vi "GPSPathTrackerTest.vi"() -> ()   [LabVIEW 2024]
uses:
  <vilib>/Instr/_visa.llb/VISA Set IO Buffer Mask.ctl
  <vilib>/Instr/_visa.llb/VISA Flush IO Buffer Mask.ctl
  <vilib>/Utility/file.llb/Read Delimited Spreadsheet (DBL).vi
  <vilib>/Instr/_visa.llb/VISA Configure Serial Port (Instr).vi
panel:
  out "True_Heading(deg)":dbl format="%#_15g"
  out "UTM X(E) INS":dbl format="%#_13g"
  out "UTM Y(N) INS":dbl format="%#_13g"
  out "GPS_Speed(kph)":dbl format="%#_g kph"
  in  "Stop":bool
  out "NMEA_Raw_Data":string
  out "Latitude(deg)":dbl
  out "Logitude(deg)":dbl
  out "Altitude(m)":dbl
  in  "COM7":refnum<visa-resource-name>="COM3" caption="GPS_Com."
  out "Path_lat_arr":dbl[](array[numeric])=[250246.8301, 250246.6716, 250246.4873, 250246.296, 250246.122, 250245.9257, 250245.7732, 250245.5875, 250245.3989, 250245.2166, 250245.0276, 250244.8653, 250244.6749, 250244.5098, 250244.319, 250244.1293, 250243.9404, 250243.757, 250243.5653, 250243.3909, 250243.2171, 250243.0265, 250242.8469, 250242.6561, 250242.4779, 250242.2931, 250242.1112, 250241.9363, 250241.7611, 250241.5908]
  out "Path_long_arr":dbl[](array[numeric])=[3688223.612, 3688223.681, 3688223.731, 3688223.77, 3688223.796, 3688223.82, 3688223.842, 3688223.793, 3688223.791, 3688223.745, 3688223.702, 3688223.665, 3688223.63, 3688223.575, 3688223.538, 3688223.496, 3688223.445, 3688223.39, 3688223.345, 3688223.293, 3688223.242, 3688223.21, 3688223.151, 3688223.108, 3688223.058, 3688223.007, 3688222.954, 3688222.905, 3688222.836, 3688222.787]
  out "Path_Vel_arr":dbl[](array[numeric])=[126.3175841, 126.3175824, 126.3175804, 126.3175784, 126.3175765, 126.3175744, 126.3175727, 126.3175708, 126.3175687, 126.3175668, 126.3175648, 126.3175631, 126.317561, 126.3175593, 126.3175572, 126.3175552, 126.3175532, 126.3175512, 126.3175492, 126.3175473, 126.3175455, 126.3175434, 126.3175415, 126.3175395, 126.3175376, 126.3175356, 126.3175337, 126.3175318, 126.31753, 126.3175282]
  out "Path_Evt_arr":dbl[](array[numeric])=[33.30420584, 33.30420642, 33.30420683, 33.30420714, 33.30420733, 33.3042075, 33.30420766, 33.30420718, 33.30420712, 33.30420667, 33.30420623, 33.30420586, 33.3042055, 33.30420497, 33.30420459, 33.30420417, 33.30420367, 33.30420313, 33.30420267, 33.30420217, 33.30420167, 33.30420133, 33.30420076, 33.30420033, 33.30419983, 33.30419933, 33.30419882, 33.30419833, 33.30419768, 33.30419719]
  out "Evt":dbl
  out "X_lat_path_Full":dbl[](array[numeric])=[250204.6315, 250204.7847, 250204.9423, 250205.0812, 250205.2434, 250205.3871, 250205.5336, 250205.6795, 250205.8333, 250205.974, 250206.1254, 250206.2733, 250206.4155, 250206.5694, 250206.7606, 250206.9331, 250207.0915, 250207.2338, 250207.3801, 250207.5358, 250207.6911, 250207.8385, 250207.9859, 250208.1346, 250208.2889, 250208.4191, 250208.562, 250208.7088, 250208.8428, 250208.9854, 250209.1251, 250209.2579, 250209.3978, 250209.5384, 250209.6838, 250209.8317, 250209.9732, 250210.1069, 250210.2502, 250210.372, 250210.5044, 250210.6376, 250210.7611, 250210.9066, 250211.0503, 250211.1744, 250211.309, 250211.4462, 250211.5776, 250211.7104, 250211.8353, 250211.9552, 250212.0902, 250212.213, 250212.3298, 250212.4572, 250212.5757, 250212.6937, 250212.8209, 250212.9386, 250213.0558, 250213.1735, 250213.2937, 250213.4125, 250213.5502, 250213.6657, 250213.7946, 250213.9274, 250214.0472, 250214.1724, 250214.3017, 250214.4417, 250214.5753, 250214.7017, 250214.8378, 250214.9662, 250215.0894, 250215.2277, 250215.372, 250215.5023, 250215.6465, 250215.6465, 250215.7658, 250215.8914, 250216.017, 250216.142, 250216.2785, 250216.4267, 250216.5776, 250216.7312, 250216.8879, 250217.0506, 250217.2131, 250217.3799, 250217.5426, 250217.7046, 250217.8748, 250218.0423, 250218.2058, 250218.3739, 250218.5355, 250218.7031, 250218.8647, 250219.0346, 250219.1961, 250219.3482, 250219.5145, 250219.672, 250219.8212, 250219.9767, 250220.1301, 250220.2837, 250220.4332, 250220.5777, 250220.7226, 250220.8672, 250221.0139, 250221.1635, 250221.2913, 250221.4361, 250221.5854, 250221.7202, 250221.862, 250222.0043, 250222.1442, 250222.2947, 250222.4297, 250222.5803, 250222.7124, 250222.8553, 250222.9875, 250223.1252, 250223.2779, 250223.409, 250223.5472, 250223.6863, 250223.8257, 250223.9601, 250224.1026, 250224.2408, 250224.3821, 250224.528, 250224.675, 250224.8272, 250224.9781, 250225.124, 250225.2738, 250225.4183, 250225.5696, 250225.7148, 250225.8666, 250226.0158, 250226.1696, 250226.314, 250226.464, 250226.616, 250226.7669, 250226.8995, 250227.0551, 250227.2017, 250227.3491, 250227.4987, 250227.651, 250227.8032, 250227.9491, 250228.1012, 250228.2468, 250228.3977, 250228.5421, 250228.6906, 250228.8411, 250228.9881, 250229.1171, 250229.2733, 250229.4177, 250229.5665, 250229.7135, 250229.8553, 250229.9955, 250230.1399, 250230.2778, 250230.4184, 250230.5592, 250230.6982, 250230.8426, 250230.9741, 250231.1183, 250231.2583, 250231.3917, 250231.5316, 250231.664, 250231.809, 250231.9365, 250232.0794, 250232.2326, 250232.3781, 250232.5288, 250232.6849, 250232.849, 250233.0169, 250233.1898, 250233.3618, 250233.5347, 250233.7129, 250233.8854, 250234.0582, 250234.2271, 250234.392, 250234.5465, 250234.6882, 250234.8252, 250234.962, 250235.0951, 250235.2304, 250235.3491, 250235.4717, 250235.6036, 250235.7176, 250235.8287, 250235.9455, 250236.054, 250236.1492, 250236.2337, 250236.312, 250236.3794, 250236.4369, 250236.4842, 250236.5555, 250236.5952, 250236.6264, 250236.6586, 250236.6755, 250236.6895, 250236.6942, 250236.697, 250236.6851, 250236.6654, 250236.6292, 250236.5933, 250236.551, 250236.4843, 250236.4291, 250236.3642, 250236.3049, 250236.2381, 250236.1715, 250236.0948, 250236.0356, 250235.9406, 250235.8714, 250235.7898, 250235.7058, 250235.658, 250235.5758, 250235.4943, 250235.4193, 250235.3767, 250235.3402, 250235.2889, 250235.2668, 250235.2332, 250235.1891, 250235.1614, 250235.1565, 250235.1204, 250235.1167, 250235.133, 250235.1628, 250235.1974, 250235.2612, 250235.3531, 250235.4155, 250235.5356, 250235.6584, 250235.7924, 250235.9326, 250236.0835, 250236.1855, 250236.3061, 250236.46, 250236.5583, 250236.7204, 250236.8858, 250237.0619, 250237.2443, 250237.4126, 250237.579, 250237.7347, 250237.9052, 250238.0628, 250238.1948, 250238.3334, 250238.4969, 250238.6626, 250238.831, 250239.0118, 250239.1778, 250239.3373, 250239.5311, 250239.6876, 250239.8513, 250240.05, 250240.2334, 250240.4321, 250240.6256, 250240.816, 250240.9998, 250241.1899, 250241.3681, 250241.5524, 250241.7339, 250241.9189, 250242.1048, 250242.2826, 250242.4514, 250242.6353, 250242.8115, 250242.986, 250243.1671, 250243.3465, 250243.5187, 250243.6972, 250243.888, 250244.084, 250244.2833, 250244.4766, 250244.6711, 250244.8658, 250245.0556, 250245.2439, 250245.4299, 250245.6119, 250245.7785, 250245.9451, 250246.096, 250246.2496, 250246.3875, 250246.5144, 250246.631, 250246.7342, 250246.8204, 250246.907, 250247.0092, 250247.1016, 250247.193, 250247.2639, 250247.3441, 250247.421, 250247.4764, 250247.5347, 250247.5768, 250247.6199, 250247.652, 250247.665, 250247.6714, 250247.6666, 250247.6394, 250247.6096, 250247.5413, 250247.498, 250247.4546, 250247.3884, 250247.3334, 250247.2883, 250247.2288, 250247.1836, 250247.1639, 250247.1466, 250247.1079, 250247.1021, 250247.0827, 250247.0531, 250247.0114, 250247.0067, 250246.9862, 250246.9811, 250246.9938, 250247.0308, 250247.0702, 250247.135, 250247.2146, 250247.3014, 250247.4225, 250247.5588, 250247.6858, 250247.828, 250247.9565, 250248.126, 250248.2664, 250248.409, 250248.5611, 250248.7068, 250248.8531, 250249.0229, 250249.202, 250249.3857, 250249.5753, 250249.7637, 250249.959, 250250.1426, 250250.3367, 250250.5143, 250250.6887, 250250.882, 250251.0751, 250251.2683, 250251.4599, 250251.6407, 250251.8269, 250252.0222, 250252.215, 250252.3883, 250252.58, 250252.7757, 250252.9624, 250253.1529, 250253.3403, 250253.5294, 250253.7184, 250253.907, 250254.0796, 250254.2588, 250254.4147, 250254.5819, 250254.743, 250254.8895, 250255.0112, 250255.1568, 250255.2877, 250255.437, 250255.5889, 250255.7462, 250255.9147, 250256.0842, 250256.2597, 250256.4476, 250256.6251, 250256.814, 250257.0016, 250257.1907, 250257.383, 250257.5732, 250257.7644, 250257.9556, 250258.1438, 250258.3228, 250258.5095, 250258.6883, 250258.8678, 250259.0368, 250259.2086, 250259.3646, 250259.5205, 250259.6669, 250259.7981, 250259.9204, 250260.0341, 250260.1304, 250260.2154, 250260.2683, 250260.3212, 250260.3713, 250260.4074, 250260.4278, 250260.4483, 250260.4538, 250260.4584, 250260.4638, 250260.4531, 250260.4269, 250260.4025, 250260.3748, 250260.3569, 250260.3259, 250260.306, 250260.3019, 250260.2913, 250260.2964, 250260.3013, 250260.322, 250260.3442, 250260.3803, 250260.414, 250260.462, 250260.5251, 250260.6072, 250260.6942, 250260.7672, 250260.8711, 250260.9697, 250261.0724, 250261.1817, 250261.2963, 250261.3941, 250261.4821, 250261.569, 250261.6706, 250261.7652, 250261.857, 250261.9183, 250261.9427, 250261.9912, 250261.9961, 250262.0007, 250261.9756, 250261.9489, 250261.9099, 250261.8812, 250261.8445, 250261.7817, 250261.7129, 250261.6398, 250261.5329, 250261.4604, 250261.3434, 250261.24, 250261.1259, 250260.9928, 250260.8741, 250260.7678, 250260.6137, 250260.4623, 250260.2939, 250260.126, 250259.9411, 250259.7546, 250259.5669, 250259.4199, 250259.2239, 250259.0425, 250258.8499, 250258.6584, 250258.475, 250258.2939, 250258.1037, 250257.9137, 250257.7231, 250257.5553, 250257.3716, 250257.2069, 250257.0301, 250256.8666, 250256.6854, 250256.514, 250256.3482, 250256.1782, 250256.0288, 250255.8463, 250255.6842, 250255.5166, 250255.3463, 250255.1982, 250255.0421, 250254.892, 250254.7261, 250254.5713, 250254.4091, 250254.2573, 250254.0995, 250253.9355, 250253.7624, 250253.5867, 250253.3985, 250253.2139, 250253.0287, 250252.8354, 250252.6448, 250252.4492, 250252.2513, 250252.0571, 250251.8685, 250251.6866, 250251.5105, 250251.3443, 250251.1824, 250251.0309, 250250.8789, 250250.7367, 250250.5995, 250250.4539, 250250.3121, 250250.1719, 250250.0299, 250249.887, 250249.7463, 250249.6052, 250249.4649, 250249.331, 250249.1893, 250249.0528, 250248.9386, 250248.8243, 250248.7236, 250248.6306, 250248.529, 250248.4359, 250248.3517, 250248.2827, 250248.2037, 250248.1463, 250248.0957, 250248.0509, 250248.0219, 250248.0051, 250247.9945, 250247.9837, 250247.989, 250247.9941, 250247.9993, 250248.0044, 250248.0095, 250248.0145, 250248.0352, 250248.0557, 250248.0919, 250248.1148, 250248.1615, 250248.1868, 250248.2214, 250248.2728, 250248.3179, 250248.3416, 250248.3511, 250248.3839, 250248.4042, 250248.432, 250248.4459, 250248.4908, 250248.5037, 250248.5435, 250248.5875, 250248.6237, 250248.6436, 250248.6662, 250248.6992, 250248.705, 250248.7258, 250248.7267, 250248.7214, 250248.7308, 250248.744, 250248.7337, 250248.7226, 250248.6855, 250248.6674, 250248.5843, 250248.537, 250248.448, 250248.3765, 250248.2712, 250248.1941, 250248.1144, 250247.9992, 250247.891, 250247.7807, 250247.6307, 250247.5171, 250247.3602, 250247.1874, 250247.0166, 250246.8301, 250246.6716, 250246.4873, 250246.296, 250246.122, 250245.9257, 250245.7732, 250245.5875, 250245.3989, 250245.2166, 250245.0276, 250244.8653, 250244.6749, 250244.5098, 250244.319, 250244.1293, 250243.9404, 250243.757, 250243.5653, 250243.3909, 250243.2171, 250243.0265, 250242.8469, 250242.6561, 250242.4779, 250242.2931, 250242.1112, 250241.9363, 250241.7611, 250241.5908, 250241.4105, 250241.2326, 250241.0415, 250240.8823, 250240.7086, 250240.5237, 250240.3385, 250240.1546, 250239.9595, 250239.7651, 250239.5694, 250239.3713, 250239.1737, 250238.9795, 250238.7874, 250238.5977, 250238.4158, 250238.2247, 250238.0451, 250237.867, 250237.6942, 250237.5189, 250237.359, 250237.1898, 250237.0315, 250236.8728, 250236.7137, 250236.5718, 250236.437, 250236.2994, 250236.1879, 250236.0639, 250235.9389, 250235.83, 250235.7229, 250235.6297, 250235.5351, 250235.4494, 250235.3697, 250235.3065, 250235.2435, 250235.1994, 250235.1375, 250235.0894, 250235.041, 250235.0127, 250234.9717, 250234.9373, 250234.9195, 250234.8912, 250234.852, 250234.8256, 250234.8066, 250234.7894, 250234.7971, 250234.798, 250234.7875, 250234.8083, 250234.8039, 250234.8027, 250234.8079, 250234.813, 250234.8181, 250234.8119, 250234.8202, 250234.8152, 250234.8222, 250234.8216, 250234.7975, 250234.7903, 250234.7485, 250234.7087, 250234.6504, 250234.616, 250234.567, 250234.5014, 250234.4497, 250234.3789, 250234.3334, 250234.2602, 250234.1655, 250234.0706, 250233.9596, 250233.8482, 250233.6928, 250233.5374, 250233.4092, 250233.2698, 250233.1115, 250232.9573, 250232.785, 250232.598, 250232.4051, 250232.2295, 250232.0509, 250231.866, 250231.6857, 250231.4995, 250231.3134, 250231.1433, 250230.9457, 250230.7492, 250230.5768, 250230.3831, 250230.1894, 250229.9975, 250229.8111, 250229.6241, 250229.4384, 250229.2517, 250229.069, 250228.8781, 250228.6895, 250228.511, 250228.3291, 250228.1418, 250227.9599, 250227.7698, 250227.597, 250227.4079, 250227.2175, 250227.0293, 250226.8363, 250226.6397, 250226.4445, 250226.4445, 250226.3195, 250226.1946, 250226.0696, 250225.9221, 250225.7742, 250225.6168, 250225.47, 250225.3233, 250225.1765, 250225.0287, 250224.8822, 250224.7443, 250224.5996, 250224.4528, 250224.301, 250224.1558, 250224.0269, 250223.8866, 250223.7351, 250223.5855, 250223.4444, 250223.2886, 250223.148, 250223.0104, 250222.8695, 250222.7295, 250222.5838, 250222.4554, 250222.316, 250222.1912, 250222.056, 250221.9297, 250221.7922, 250221.6642, 250221.5466, 250221.3995, 250221.2768, 250221.1432, 250221.0095, 250220.8891, 250220.7597, 250220.6502, 250220.5287, 250220.4116, 250220.2851, 250220.1647, 250220.0444, 250219.9261, 250219.7966, 250219.6741, 250219.5628, 250219.4354, 250219.3182, 250219.1887, 250219.0582, 250218.9251, 250218.8036, 250218.679, 250218.5495, 250218.4169, 250218.2866, 250218.1513, 250218.0199, 250217.8896, 250217.7568, 250217.6185, 250217.4845, 250217.3551, 250217.2166, 250217.0853, 250216.9453, 250216.8055, 250216.6585, 250216.5131, 250216.3689, 250216.2118, 250216.0655, 250215.9129, 250215.7606, 250215.6071, 250215.4505, 250215.2942, 250215.1411, 250214.9841, 250214.842, 250214.6871, 250214.5483, 250214.3987, 250214.2557, 250214.1195, 250213.9747, 250213.8377, 250213.7044, 250213.5703, 250213.4445, 250213.3184, 250213.183, 250213.0559, 250212.9317, 250212.8112, 250212.6789, 250212.5512, 250212.4267, 250212.2918, 250212.1645, 250212.0429, 250211.9046, 250211.769, 250211.6308, 250211.492, 250211.3609, 250211.2259, 250211.0952, 250210.9578, 250210.8141, 250210.6818, 250210.5388, 250210.4096, 250210.2669, 250210.1265, 250209.986, 250209.8443, 250209.696, 250209.5582, 250209.4275, 250209.2882, 250209.1319, 250209.0284]
  out "vel. path":dbl[](array[numeric])=[126.317125, 126.3171267, 126.3171284, 126.3171299, 126.3171317, 126.3171333, 126.3171349, 126.3171365, 126.3171382, 126.3171397, 126.3171414, 126.317143, 126.3171446, 126.3171463, 126.3171483, 126.3171502, 126.317152, 126.3171535, 126.3171551, 126.3171568, 126.3171585, 126.3171601, 126.3171618, 126.3171634, 126.3171651, 126.3171665, 126.3171681, 126.3171697, 126.3171712, 126.3171728, 126.3171743, 126.3171758, 126.3171773, 126.3171788, 126.3171804, 126.3171821, 126.3171836, 126.3171851, 126.3171867, 126.317188, 126.3171895, 126.317191, 126.3171923, 126.3171939, 126.3171955, 126.3171969, 126.3171984, 126.3171999, 126.3172013, 126.3172028, 126.3172042, 126.3172055, 126.317207, 126.3172083, 126.3172096, 126.3172111, 126.3172124, 126.3172137, 126.3172151, 126.3172164, 126.3172177, 126.317219, 126.3172203, 126.3172217, 126.3172232, 126.3172245, 126.3172259, 126.3172273, 126.3172287, 126.3172301, 126.3172315, 126.317233, 126.3172345, 126.3172359, 126.3172374, 126.3172388, 126.3172402, 126.3172417, 126.3172433, 126.3172447, 126.3172463, 126.3172463, 126.3172476, 126.317249, 126.3172504, 126.3172518, 126.3172533, 126.3172549, 126.3172566, 126.3172583, 126.31726, 126.3172618, 126.3172635, 126.3172654, 126.3172671, 126.3172689, 126.3172708, 126.3172726, 126.3172744, 126.3172762, 126.317278, 126.3172798, 126.3172816, 126.3172834, 126.3172852, 126.3172868, 126.3172886, 126.3172904, 126.317292, 126.3172937, 126.3172954, 126.3172971, 126.3172987, 126.3173003, 126.3173019, 126.3173035, 126.3173051, 126.3173067, 126.3173081, 126.3173097, 126.3173114, 126.3173129, 126.3173144, 126.317316, 126.3173175, 126.3173192, 126.3173207, 126.3173223, 126.3173238, 126.3173253, 126.3173268, 126.3173283, 126.31733, 126.3173314, 126.317333, 126.3173345, 126.317336, 126.3173375, 126.3173391, 126.3173406, 126.3173421, 126.3173437, 126.3173454, 126.317347, 126.3173487, 126.3173503, 126.3173519, 126.3173535, 126.3173552, 126.3173568, 126.3173584, 126.3173601, 126.3173617, 126.3173633, 126.317365, 126.3173666, 126.3173683, 126.3173698, 126.3173715, 126.3173731, 126.3173747, 126.3173763, 126.317378, 126.3173797, 126.3173813, 126.3173829, 126.3173845, 126.3173862, 126.3173878, 126.3173894, 126.3173911, 126.3173927, 126.3173941, 126.3173958, 126.3173974, 126.317399, 126.3174006, 126.3174022, 126.3174037, 126.3174053, 126.3174068, 126.3174084, 126.3174099, 126.3174115, 126.3174131, 126.3174145, 126.3174161, 126.3174176, 126.3174191, 126.3174206, 126.3174221, 126.3174237, 126.3174251, 126.3174267, 126.3174284, 126.31743, 126.3174316, 126.3174333, 126.3174351, 126.3174369, 126.3174388, 126.3174407, 126.3174426, 126.3174445, 126.3174464, 126.3174483, 126.3174501, 126.3174519, 126.3174536, 126.3174552, 126.3174567, 126.3174582, 126.3174596, 126.3174611, 126.3174624, 126.3174638, 126.3174653, 126.3174665, 126.3174678, 126.3174691, 126.3174703, 126.3174713, 126.3174723, 126.3174732, 126.317474, 126.3174746, 126.3174752, 126.317476, 126.3174765, 126.3174769, 126.3174773, 126.3174775, 126.3174777, 126.3174778, 126.3174779, 126.3174778, 126.3174777, 126.3174773, 126.317477, 126.3174766, 126.3174759, 126.3174754, 126.3174748, 126.3174742, 126.3174735, 126.3174728, 126.3174721, 126.3174715, 126.3174705, 126.3174698, 126.317469, 126.3174681, 126.3174677, 126.3174668, 126.317466, 126.3174653, 126.3174648, 126.3174645, 126.317464, 126.3174638, 126.3174635, 126.3174631, 126.3174628, 126.3174628, 126.3174625, 126.3174625, 126.3174627, 126.3174631, 126.3174635, 126.3174643, 126.3174653, 126.317466, 126.3174673, 126.3174687, 126.3174702, 126.3174717, 126.3174734, 126.3174745, 126.3174758, 126.3174775, 126.31747849999999, 126.3174803, 126.3174821, 126.317484, 126.317486, 126.3174878, 126.3174896, 126.3174913, 126.3174932, 126.3174949, 126.3174963, 126.3174978, 126.3174996, 126.3175014, 126.3175032, 126.3175052, 126.317507, 126.3175087, 126.3175108, 126.3175125, 126.3175142, 126.3175164, 126.3175183, 126.3175205, 126.3175225, 126.3175246, 126.3175265, 126.3175286, 126.3175305, 126.3175324, 126.3175344, 126.3175363, 126.3175383, 126.3175402, 126.317542, 126.3175439, 126.3175458, 126.3175477, 126.3175496, 126.3175515, 126.3175533, 126.3175552, 126.3175573, 126.3175594, 126.3175615, 126.3175636, 126.3175657, 126.3175678, 126.3175698, 126.3175719, 126.3175739, 126.3175759, 126.3175777, 126.3175795, 126.3175811, 126.3175828, 126.3175843, 126.3175857, 126.317587, 126.3175882, 126.3175892, 126.3175901, 126.3175913, 126.3175923, 126.3175933, 126.3175942, 126.3175951, 126.3175959, 126.3175966, 126.3175973, 126.3175978, 126.3175983, 126.3175987, 126.3175989, 126.317599, 126.317599, 126.3175988, 126.3175985, 126.3175978, 126.3175974, 126.317597, 126.3175963, 126.3175958, 126.3175954, 126.3175948, 126.3175943, 126.3175942, 126.317594, 126.3175937, 126.3175937, 126.3175935, 126.3175932, 126.3175928, 126.3175928, 126.3175927, 126.3175927, 126.3175929, 126.3175933, 126.3175938, 126.3175945, 126.3175954, 126.3175964, 126.3175977, 126.3175992, 126.3176006, 126.3176022, 126.3176036, 126.3176055, 126.317607, 126.3176086, 126.3176102, 126.3176118, 126.3176134, 126.3176152, 126.3176172, 126.3176192, 126.3176212, 126.3176233, 126.3176254, 126.3176274, 126.3176294, 126.3176314, 126.3176333, 126.3176353, 126.3176374, 126.3176395, 126.3176416, 126.3176435, 126.3176455, 126.3176476, 126.3176497, 126.3176515, 126.3176536, 126.3176557, 126.3176577, 126.3176597, 126.3176617, 126.3176637, 126.3176657, 126.3176677, 126.3176696, 126.3176715, 126.3176731, 126.3176749, 126.3176766, 126.3176781, 126.3176794, 126.3176809, 126.3176823, 126.3176838, 126.3176854, 126.3176871, 126.3176889, 126.3176906, 126.3176925, 126.3176945, 126.3176964, 126.3176984, 126.3177004, 126.3177024, 126.3177044, 126.3177065, 126.3177085, 126.3177106, 126.3177126, 126.3177145, 126.3177164, 126.3177183, 126.3177202, 126.317722, 126.3177238, 126.3177255, 126.3177271, 126.3177287, 126.31773, 126.3177313, 126.3177325, 126.3177335, 126.3177343, 126.3177348, 126.3177353, 126.3177358, 126.3177362, 126.3177363, 126.3177365, 126.3177365, 126.3177365, 126.3177365, 126.3177363, 126.317736, 126.3177357, 126.3177353, 126.3177351, 126.3177347, 126.3177344, 126.3177343, 126.3177342, 126.3177342, 126.3177342, 126.3177343, 126.3177345, 126.3177349, 126.3177352, 126.3177356, 126.3177362, 126.3177371, 126.317738, 126.3177387, 126.3177398, 126.3177408, 126.3177418, 126.317743, 126.3177441, 126.3177452, 126.317746, 126.3177469, 126.317748, 126.3177489, 126.3177499, 126.3177505, 126.3177507, 126.3177512, 126.3177512, 126.3177512, 126.3177508, 126.3177505, 126.31775, 126.3177497, 126.3177492, 126.3177485, 126.3177477, 126.3177469, 126.3177457, 126.3177449, 126.3177436, 126.3177424, 126.3177412, 126.3177397, 126.3177384, 126.3177372, 126.3177355, 126.3177339, 126.317732, 126.3177302, 126.3177282, 126.3177262, 126.3177242, 126.3177226, 126.3177205, 126.3177186, 126.3177165, 126.3177145, 126.3177125, 126.3177106, 126.3177085, 126.3177065, 126.3177045, 126.3177027, 126.3177007, 126.317699, 126.3176971, 126.3176954, 126.3176934, 126.3176916, 126.3176899, 126.3176881, 126.3176865, 126.3176845, 126.3176828, 126.3176811, 126.3176793, 126.3176777, 126.317676, 126.3176745, 126.3176727, 126.3176711, 126.3176694, 126.3176678, 126.3176661, 126.3176644, 126.3176626, 126.3176607, 126.3176587, 126.3176567, 126.3176548, 126.3176527, 126.3176507, 126.3176486, 126.3176464, 126.3176444, 126.3176423, 126.3176403, 126.3176384, 126.3176366, 126.3176349, 126.3176332, 126.3176315, 126.31763, 126.3176285, 126.3176269, 126.3176253, 126.3176238, 126.3176222, 126.3176206, 126.3176191, 126.3176175, 126.317616, 126.3176145, 126.3176129, 126.3176114, 126.3176102, 126.3176089, 126.3176078, 126.3176067, 126.3176056, 126.3176045, 126.3176036, 126.3176028, 126.3176019, 126.3176012, 126.3176006, 126.3176001, 126.3175997, 126.3175995, 126.3175993, 126.3175992, 126.3175992, 126.3175992, 126.3175992, 126.3175992, 126.3175992, 126.3175992, 126.3175993, 126.3175995, 126.3175998, 126.3176, 126.3176005, 126.3176007, 126.317601, 126.3176015, 126.3176019, 126.3176022, 126.3176022, 126.3176025, 126.3176027, 126.3176029, 126.317603, 126.3176034, 126.3176035, 126.3176039, 126.3176043, 126.3176047, 126.3176048, 126.317605, 126.3176053, 126.3176053, 126.3176055, 126.3176055, 126.3176054, 126.3176054, 126.3176055, 126.3176053, 126.3176052, 126.3176047, 126.3176045, 126.3176035, 126.317603, 126.317602, 126.3176012, 126.3176, 126.3175991, 126.3175982, 126.3175969, 126.3175957, 126.3175945, 126.3175929, 126.3175916, 126.3175899, 126.317588, 126.3175862, 126.3175841, 126.3175824, 126.3175804, 126.3175784, 126.3175765, 126.3175744, 126.3175727, 126.3175708, 126.3175687, 126.3175668, 126.3175648, 126.3175631, 126.317561, 126.3175593, 126.3175572, 126.3175552, 126.3175532, 126.3175512, 126.3175492, 126.3175473, 126.3175455, 126.3175434, 126.3175415, 126.3175395, 126.3175376, 126.3175356, 126.3175337, 126.3175318, 126.31753, 126.3175282, 126.3175262, 126.3175243, 126.3175223, 126.3175206, 126.3175188, 126.3175168, 126.3175148, 126.3175129, 126.3175108, 126.3175087, 126.3175066, 126.3175045, 126.3175024, 126.3175003, 126.3174982, 126.3174961, 126.3174942, 126.3174921, 126.3174902, 126.3174882, 126.3174863, 126.3174844, 126.3174827, 126.3174809, 126.3174791, 126.3174774, 126.3174756, 126.3174741, 126.3174726, 126.3174711, 126.3174698, 126.3174685, 126.3174671, 126.3174659, 126.3174647, 126.3174636, 126.3174626, 126.3174616, 126.3174607, 126.31746, 126.3174592, 126.3174587, 126.317458, 126.3174574, 126.3174568, 126.3174565, 126.317456, 126.3174556, 126.3174553, 126.317455, 126.3174545, 126.3174542, 126.3174539, 126.3174537, 126.3174537, 126.3174537, 126.3174535, 126.3174537, 126.3174536, 126.3174535, 126.3174535, 126.3174535, 126.3174535, 126.3174534, 126.3174534, 126.3174533, 126.3174533, 126.3174533, 126.317453, 126.3174528, 126.3174523, 126.3174519, 126.3174512, 126.3174508, 126.3174502, 126.3174494, 126.3174488, 126.317448, 126.3174475, 126.3174467, 126.3174456, 126.3174445, 126.3174433, 126.3174421, 126.3174404, 126.3174387, 126.3174373, 126.3174358, 126.317434, 126.3174324, 126.3174305, 126.3174285, 126.3174264, 126.3174245, 126.3174226, 126.3174206, 126.3174187, 126.3174167, 126.3174147, 126.3174128, 126.3174107, 126.3174086, 126.3174068, 126.3174047, 126.3174026, 126.3174006, 126.3173986, 126.3173966, 126.3173946, 126.3173926, 126.3173907, 126.3173887, 126.3173867, 126.3173848, 126.3173828, 126.3173808, 126.3173789, 126.3173769, 126.317375, 126.317373, 126.317371, 126.317369, 126.3173669, 126.31736480000001, 126.3173627, 126.3173627, 126.3173614, 126.31736, 126.3173587, 126.3173571, 126.3173554, 126.3173537, 126.3173521, 126.3173505, 126.3173489, 126.3173473, 126.3173457, 126.3173441, 126.3173426, 126.3173409, 126.3173393, 126.3173377, 126.3173363, 126.3173347, 126.3173331, 126.3173314, 126.3173299, 126.3173282, 126.3173266, 126.3173251, 126.3173235, 126.317322, 126.3173204, 126.317319, 126.3173175, 126.3173161, 126.3173146, 126.3173132, 126.3173117, 126.3173103, 126.3173089, 126.3173073, 126.317306, 126.3173045, 126.317303, 126.3173017, 126.3173003, 126.317299, 126.3172977, 126.3172964, 126.317295, 126.3172937, 126.3172923, 126.317291, 126.3172896, 126.3172882, 126.317287, 126.3172856, 126.3172843, 126.3172829, 126.3172814, 126.31728, 126.3172786, 126.3172772, 126.3172758, 126.3172743, 126.3172729, 126.3172714, 126.31727, 126.3172685, 126.317267, 126.3172655, 126.317264, 126.3172626, 126.3172611, 126.3172596, 126.3172581, 126.3172566, 126.317255, 126.3172534, 126.3172518, 126.3172501, 126.3172485, 126.3172468, 126.3172451, 126.3172434, 126.3172417, 126.31724, 126.3172383, 126.3172366, 126.3172351, 126.3172334, 126.3172318, 126.3172302, 126.3172286, 126.3172271, 126.3172255, 126.317224, 126.3172225, 126.3172211, 126.3172197, 126.3172183, 126.3172168, 126.3172154, 126.317214, 126.3172127, 126.3172112, 126.3172098, 126.3172084, 126.3172069, 126.3172055, 126.3172042, 126.3172027, 126.3172012, 126.3171997, 126.3171981, 126.3171967, 126.3171952, 126.3171937, 126.3171922, 126.3171907, 126.3171892, 126.3171876, 126.3171862, 126.3171846, 126.3171831, 126.3171815, 126.31718, 126.3171783, 126.3171768, 126.3171754, 126.3171739, 126.3171721, 126.317171]
  out "Y_long_path_Full":dbl[](array[numeric])=[3688246.636, 3688246.509, 3688246.386, 3688246.252, 3688246.131, 3688245.999, 3688245.863, 3688245.725, 3688245.593, 3688245.45, 3688245.315, 3688245.179, 3688245.039, 3688244.911, 3688244.843, 3688244.735, 3688244.608, 3688244.485, 3688244.347, 3688244.225, 3688244.098, 3688243.962, 3688243.826, 3688243.702, 3688243.576, 3688243.428, 3688243.289, 3688243.152, 3688243.019, 3688242.881, 3688242.758, 3688242.611, 3688242.466, 3688242.324, 3688242.184, 3688242.046, 3688241.912, 3688241.761, 3688241.621, 3688241.464, 3688241.317, 3688241.168, 3688241.016, 3688240.878, 3688240.743, 3688240.587, 3688240.445, 3688240.302, 3688240.154, 3688240.007, 3688239.85, 3688239.697, 3688239.549, 3688239.391, 3688239.229, 3688239.078, 3688238.919, 3688238.759, 3688238.606, 3688238.449, 3688238.288, 3688238.132, 3688237.972, 3688237.812, 3688237.667, 3688237.509, 3688237.359, 3688237.212, 3688237.056, 3688236.903, 3688236.761, 3688236.618, 3688236.472, 3688236.318, 3688236.18, 3688236.04, 3688235.882, 3688235.736, 3688235.602, 3688235.455, 3688235.317, 3688235.317, 3688235.161, 3688235.009, 3688234.859, 3688234.707, 3688234.563, 3688234.431, 3688234.301, 3688234.177, 3688234.058, 3688233.945, 3688233.832, 3688233.726, 3688233.616, 3688233.504, 3688233.406, 3688233.302, 3688233.192, 3688233.09, 3688232.98, 3688232.875, 3688232.767, 3688232.663, 3688232.554, 3688232.429, 3688232.322, 3688232.207, 3688232.075, 3688231.951, 3688231.826, 3688231.702, 3688231.575, 3688231.444, 3688231.311, 3688231.182, 3688231.047, 3688230.919, 3688230.774, 3688230.641, 3688230.511, 3688230.367, 3688230.231, 3688230.094, 3688229.957, 3688229.829, 3688229.683, 3688229.557, 3688229.413, 3688229.278, 3688229.132, 3688228.991, 3688228.865, 3688228.717, 3688228.577, 3688228.436, 3688228.296, 3688228.16, 3688228.023, 3688227.884, 3688227.749, 3688227.618, 3688227.486, 3688227.365, 3688227.239, 3688227.103, 3688226.975, 3688226.839, 3688226.711, 3688226.574, 3688226.45, 3688226.318, 3688226.199, 3688226.063, 3688225.934, 3688225.812, 3688225.684, 3688225.54, 3688225.421, 3688225.29, 3688225.156, 3688225.028, 3688224.9, 3688224.772, 3688224.642, 3688224.516, 3688224.383, 3688224.257, 3688224.124, 3688223.994, 3688223.865, 3688223.735, 3688223.59, 3688223.474, 3688223.338, 3688223.207, 3688223.074, 3688222.936, 3688222.795, 3688222.659, 3688222.518, 3688222.382, 3688222.244, 3688222.105, 3688221.97, 3688221.825, 3688221.694, 3688221.554, 3688221.407, 3688221.266, 3688221.121, 3688220.986, 3688220.837, 3688220.7, 3688220.579, 3688220.446, 3688220.321, 3688220.2, 3688220.09, 3688219.984, 3688219.886, 3688219.791, 3688219.695, 3688219.609, 3688219.511, 3688219.412, 3688219.312, 3688219.202, 3688219.08, 3688218.943, 3688218.802, 3688218.658, 3688218.514, 3688218.373, 3688218.215, 3688218.06, 3688217.916, 3688217.752, 3688217.592, 3688217.434, 3688217.271, 3688217.096, 3688216.918, 3688216.738, 3688216.555, 3688216.364, 3688216.175, 3688215.99, 3688215.797, 3688215.603, 3688215.408, 3688215.212, 3688215.018, 3688214.825, 3688214.629, 3688214.435, 3688214.238, 3688214.045, 3688213.854, 3688213.659, 3688213.473, 3688213.282, 3688213.096, 3688212.911, 3688212.732, 3688212.553, 3688212.373, 3688212.187, 3688212.026, 3688211.845, 3688211.666, 3688211.498, 3688211.307, 3688211.137, 3688210.957, 3688210.774, 3688210.583, 3688210.455, 3688210.27, 3688210.079, 3688209.89, 3688209.707, 3688209.511, 3688209.32, 3688209.133, 3688208.944, 3688208.778, 3688208.603, 3688208.425, 3688208.24, 3688208.069, 3688207.923, 3688207.776, 3688207.638, 3688207.505, 3688207.376, 3688207.261, 3688207.163, 3688207.105, 3688206.993, 3688206.89, 3688206.843, 3688206.777, 3688206.715, 3688206.655, 3688206.559, 3688206.461, 3688206.366, 3688206.273, 3688206.184, 3688206.113, 3688205.99, 3688205.895, 3688205.827, 3688205.775, 3688205.706, 3688205.658, 3688205.603, 3688205.616, 3688205.607, 3688205.608, 3688205.602, 3688205.579, 3688205.574, 3688205.595, 3688205.626, 3688205.67, 3688205.702, 3688205.765, 3688205.832, 3688205.892, 3688205.924, 3688205.975, 3688206.044, 3688206.125, 3688206.183, 3688206.249, 3688206.333, 3688206.409, 3688206.446, 3688206.526, 3688206.566, 3688206.595, 3688206.609, 3688206.603, 3688206.58, 3688206.556, 3688206.533, 3688206.491, 3688206.441, 3688206.381, 3688206.31, 3688206.213, 3688206.118, 3688205.996, 3688205.876, 3688205.735, 3688205.585, 3688205.428, 3688205.261, 3688205.087, 3688204.913, 3688204.745, 3688204.572, 3688204.399, 3688204.217, 3688204.041, 3688203.86, 3688203.671, 3688203.482, 3688203.291, 3688203.097, 3688202.903, 3688202.706, 3688202.51, 3688202.313, 3688202.121, 3688201.928, 3688201.742, 3688201.55, 3688201.357, 3688201.175, 3688201.009, 3688200.831, 3688200.66, 3688200.469, 3688200.293, 3688200.102, 3688199.927, 3688199.75, 3688199.553, 3688199.364, 3688199.207, 3688199.015, 3688198.819, 3688198.62, 3688198.43, 3688198.239, 3688198.051, 3688197.866, 3688197.706, 3688197.53, 3688197.389, 3688197.254, 3688197.113, 3688197.004, 3688196.877, 3688196.777, 3688196.671, 3688196.564, 3688196.467, 3688196.356, 3688196.256, 3688196.178, 3688196.107, 3688196.03, 3688195.977, 3688195.933, 3688195.904, 3688195.84, 3688195.809, 3688195.77, 3688195.714, 3688195.686, 3688195.663, 3688195.635, 3688195.597, 3688195.593, 3688195.569, 3688195.582, 3688195.578, 3688195.592, 3688195.622, 3688195.638, 3688195.688, 3688195.721, 3688195.771, 3688195.83, 3688195.888, 3688195.924, 3688196.013, 3688196.097, 3688196.199, 3688196.297, 3688196.407, 3688196.538, 3688196.689, 3688196.822, 3688196.969, 3688197.098, 3688197.223, 3688197.336, 3688197.437, 3688197.537, 3688197.627, 3688197.689, 3688197.772, 3688197.835, 3688197.898, 3688197.962, 3688198.006, 3688198.066, 3688198.118, 3688198.16, 3688198.22, 3688198.3, 3688198.363, 3688198.445, 3688198.523, 3688198.622, 3688198.722, 3688198.834, 3688198.951, 3688199.084, 3688199.233, 3688199.389, 3688199.552, 3688199.724, 3688199.899, 3688200.09, 3688200.276, 3688200.466, 3688200.659, 3688200.855, 3688201.049, 3688201.243, 3688201.442, 3688201.641, 3688201.837, 3688202.031, 3688202.224, 3688202.419, 3688202.615, 3688202.809, 3688203.003, 3688203.2, 3688203.398, 3688203.596, 3688203.795, 3688203.99, 3688204.187, 3688204.382, 3688204.576, 3688204.768, 3688204.955, 3688205.134, 3688205.302, 3688205.48, 3688205.649, 3688205.819, 3688205.987, 3688206.153, 3688206.315, 3688206.475, 3688206.647, 3688206.821, 3688206.984, 3688207.155, 3688207.331, 3688207.516, 3688207.707, 3688207.883, 3688208.081, 3688208.28, 3688208.475, 3688208.668, 3688208.858, 3688209.044, 3688209.226, 3688209.406, 3688209.585, 3688209.736, 3688209.892, 3688210.061, 3688210.21, 3688210.376, 3688210.537, 3688210.657, 3688210.774, 3688210.911, 3688211.029, 3688211.149, 3688211.236, 3688211.32, 3688211.383, 3688211.44, 3688211.445, 3688211.43, 3688211.417, 3688211.403, 3688211.371, 3688211.339, 3688211.288, 3688211.266, 3688211.231, 3688211.192, 3688211.159, 3688211.09, 3688211.04, 3688210.987, 3688210.902, 3688210.837, 3688210.775, 3688210.694, 3688210.621, 3688210.559, 3688210.478, 3688210.405, 3688210.295, 3688210.196, 3688210.103, 3688209.986, 3688209.897, 3688209.77, 3688209.673, 3688209.572, 3688209.462, 3688209.359, 3688209.244, 3688209.133, 3688209.036, 3688208.949, 3688208.891, 3688208.817, 3688208.749, 3688208.713, 3688208.664, 3688208.65, 3688208.66, 3688208.683, 3688208.737, 3688208.812, 3688208.9, 3688209.001, 3688209.113, 3688209.24, 3688209.367, 3688209.505, 3688209.64, 3688209.773, 3688209.904, 3688210.04, 3688210.178, 3688210.315, 3688210.453, 3688210.59, 3688210.727, 3688210.871, 3688211.008, 3688211.148, 3688211.311, 3688211.471, 3688211.642, 3688211.815, 3688211.983, 3688212.159, 3688212.339, 3688212.521, 3688212.701, 3688212.891, 3688213.083, 3688213.276, 3688213.469, 3688213.666, 3688213.862, 3688214.057, 3688214.255, 3688214.453, 3688214.653, 3688214.853, 3688215.051, 3688215.25, 3688215.444, 3688215.641, 3688215.834, 3688216.03, 3688216.22, 3688216.415, 3688216.609, 3688216.798, 3688216.975, 3688217.146, 3688217.341, 3688217.523, 3688217.718, 3688217.904, 3688218.088, 3688218.264, 3688218.452, 3688218.624, 3688218.803, 3688218.991, 3688219.18, 3688219.365, 3688219.554, 3688219.748, 3688219.937, 3688220.115, 3688220.312, 3688220.462, 3688220.658, 3688220.856, 3688221.033, 3688221.218, 3688221.387, 3688221.55, 3688221.723, 3688221.888, 3688222.066, 3688222.206, 3688222.378, 3688222.54, 3688222.688, 3688222.84, 3688222.985, 3688223.105, 3688223.246, 3688223.363, 3688223.459, 3688223.551, 3688223.612, 3688223.681, 3688223.731, 3688223.77, 3688223.796, 3688223.82, 3688223.842, 3688223.793, 3688223.791, 3688223.745, 3688223.702, 3688223.665, 3688223.63, 3688223.575, 3688223.538, 3688223.496, 3688223.445, 3688223.39, 3688223.345, 3688223.293, 3688223.242, 3688223.21, 3688223.151, 3688223.108, 3688223.058, 3688223.007, 3688222.954, 3688222.905, 3688222.836, 3688222.787, 3688222.74, 3688222.683, 3688222.638, 3688222.586, 3688222.511, 3688222.478, 3688222.412, 3688222.359, 3688222.34, 3688222.314, 3688222.3, 3688222.305, 3688222.31, 3688222.337, 3688222.376, 3688222.424, 3688222.483, 3688222.527, 3688222.608, 3688222.689, 3688222.783, 3688222.873, 3688222.992, 3688223.093, 3688223.213, 3688223.334, 3688223.454, 3688223.591, 3688223.737, 3688223.876, 3688224.034, 3688224.188, 3688224.344, 3688224.508, 3688224.673, 3688224.847, 3688225.02, 3688225.2, 3688225.381, 3688225.567, 3688225.754, 3688225.947, 3688226.135, 3688226.326, 3688226.518, 3688226.714, 3688226.903, 3688227.091, 3688227.284, 3688227.478, 3688227.672, 3688227.866, 3688228.052, 3688228.244, 3688228.437, 3688228.601, 3688228.797, 3688228.994, 3688229.189, 3688229.387, 3688229.587, 3688229.785, 3688229.985, 3688230.183, 3688230.38, 3688230.566, 3688230.748, 3688230.94, 3688231.128, 3688231.318, 3688231.504, 3688231.693, 3688231.866, 3688232.053, 3688232.23, 3688232.388, 3688232.573, 3688232.725, 3688232.88, 3688233.054, 3688233.218, 3688233.39, 3688233.528, 3688233.686, 3688233.804, 3688233.914, 3688234.006, 3688234.079, 3688234.157, 3688234.233, 3688234.306, 3688234.361, 3688234.397, 3688234.42, 3688234.426, 3688234.413, 3688234.415, 3688234.412, 3688234.395, 3688234.411, 3688234.397, 3688234.384, 3688234.363, 3688234.325, 3688234.303, 3688234.255, 3688234.209, 3688234.17, 3688234.122, 3688234.08, 3688234.02, 3688233.976, 3688233.93, 3688233.866, 3688233.809, 3688233.757, 3688233.697, 3688233.665, 3688233.601, 3688233.564, 3688233.533, 3688233.503, 3688233.455, 3688233.435, 3688233.422, 3688233.422, 3688233.413, 3688233.405, 3688233.397, 3688233.525, 3688233.659, 3688233.778, 3688233.911, 3688234.043, 3688234.174, 3688234.307, 3688234.435, 3688234.569, 3688234.705, 3688234.84, 3688234.961, 3688235.097, 3688235.227, 3688235.365, 3688235.493, 3688235.623, 3688235.758, 3688235.877, 3688236.014, 3688236.159, 3688236.295, 3688236.435, 3688236.571, 3688236.724, 3688236.867, 3688237.018, 3688237.158, 3688237.308, 3688237.453, 3688237.606, 3688237.764, 3688237.899, 3688238.054, 3688238.201, 3688238.349, 3688238.502, 3688238.644, 3688238.795, 3688238.953, 3688239.112, 3688239.259, 3688239.41, 3688239.562, 3688239.702, 3688239.853, 3688240.006, 3688240.166, 3688240.313, 3688240.473, 3688240.61, 3688240.762, 3688240.907, 3688241.061, 3688241.213, 3688241.362, 3688241.508, 3688241.659, 3688241.804, 3688241.946, 3688242.094, 3688242.243, 3688242.387, 3688242.527, 3688242.67, 3688242.808, 3688242.951, 3688243.091, 3688243.229, 3688243.354, 3688243.482, 3688243.612, 3688243.732, 3688243.857, 3688243.981, 3688244.094, 3688244.219, 3688244.343, 3688244.466, 3688244.587, 3688244.708, 3688244.84, 3688244.965, 3688245.103, 3688245.229, 3688245.362, 3688245.503, 3688245.64, 3688245.78, 3688245.922, 3688246.064, 3688246.214, 3688246.361, 3688246.508, 3688246.655, 3688246.809, 3688246.962, 3688247.108, 3688247.256, 3688247.407, 3688247.548, 3688247.695, 3688247.846, 3688247.99, 3688248.13, 3688248.271, 3688248.412, 3688248.553, 3688248.699, 3688248.848, 3688248.992, 3688249.128, 3688249.276, 3688249.41, 3688249.556, 3688249.69, 3688249.832, 3688249.967, 3688250.104, 3688250.232, 3688250.375, 3688250.521, 3688250.658, 3688250.777, 3688250.901]
  out "Evt.Arr":dbl[](array[numeric])=[33.3044035, 33.3044024, 33.30440132, 33.30440015, 33.3043991, 33.30439794, 33.30439675, 33.30439554, 33.30439439, 33.30439313, 33.30439195, 33.30439076, 33.30438953, 33.30438841, 33.30438784, 33.30438692, 33.3043858, 33.30438473, 33.30438352, 33.30438245, 33.30438134, 33.30438015, 33.30437896, 33.30437788, 33.30437678, 33.30437548, 33.30437425, 33.30437306, 33.30437189, 33.30437068, 33.3043696, 33.30436831, 33.30436703, 33.30436578, 33.30436456, 33.30436336, 33.30436217, 33.30436085, 33.30435962, 33.30435823, 33.30435694, 33.30435563, 33.30435428, 33.30435308, 33.30435189, 33.30435052, 33.30434926, 33.30434801, 33.30434672, 33.30434541, 33.30434403, 33.30434268, 33.30434137, 33.30433998, 33.30433855, 33.30433722, 33.30433581, 33.3043344, 33.30433306, 33.30433166, 33.30433024, 33.30432886, 33.30432745, 33.30432603, 33.30432476, 33.30432336, 33.30432204, 33.30432075, 33.30431937, 33.30431801, 33.30431677, 33.30431551, 33.30431422, 33.30431287, 33.30431166, 33.30431043, 33.30430903, 33.30430775, 33.30430658, 33.30430528, 33.30430407, 33.30430407, 33.30430269, 33.30430135, 33.30430003, 33.30429869, 33.30429743, 33.30429627, 33.30429513, 33.30429405, 33.30429302, 33.30429204, 33.30429106, 33.30429014, 33.30428918, 33.30428821, 33.30428737, 33.30428647, 33.30428552, 33.30428464, 33.30428368, 33.30428278, 33.30428184, 33.30428095, 33.30428, 33.30427891, 33.30427798, 33.30427698, 33.30427583, 33.30427475, 33.30427366, 33.30427257, 33.30427147, 33.30427032, 33.30426916, 33.30426802, 33.30426685, 33.30426572, 33.30426445, 33.30426329, 33.30426215, 33.30426088, 33.30425969, 33.30425848, 33.30425728, 33.30425617, 33.30425488, 33.30425379, 33.30425252, 33.30425133, 33.30425005, 33.30424881, 33.30424771, 33.3042464, 33.30424517, 33.30424394, 33.30424271, 33.30424152, 33.30424032, 33.30423909, 33.30423791, 33.30423676, 33.30423561, 33.30423456, 33.30423346, 33.30423226, 33.30423114, 33.30422995, 33.30422883, 33.30422763, 33.30422655, 33.3042254, 33.30422436, 33.30422317, 33.30422204, 33.30422098, 33.30421986, 33.30421859, 33.30421756, 33.30421641, 33.30421523, 33.30421412, 33.304213, 33.30421188, 33.30421074, 33.30420964, 33.30420848, 33.30420738, 33.30420621, 33.30420507, 33.30420395, 33.30420281, 33.30420153, 33.30420052, 33.30419933, 33.30419819, 33.30419702, 33.30419581, 33.30419457, 33.30419338, 33.30419214, 33.30419095, 33.30418974, 33.30418852, 33.30418734, 33.30418606, 33.30418491, 33.30418369, 33.3041824, 33.30418115, 33.30417988, 33.30417869, 33.30417738, 33.30417618, 33.30417512, 33.30417397, 33.30417287, 33.30417182, 33.30417087, 33.30416994, 33.3041691, 33.30416829, 33.30416747, 33.30416673, 33.30416589, 33.30416503, 33.30416417, 33.30416322, 33.30416216, 33.30416095, 33.30415971, 33.30415845, 33.30415719, 33.30415595, 33.30415455, 33.30415318, 33.30415192, 33.30415047, 33.30414905, 33.30414765, 33.30414621, 33.30414465, 33.30414307, 33.30414146, 33.30413983, 33.30413813, 33.30413643, 33.30413478, 33.30413306, 33.30413131, 33.30412956, 33.3041278, 33.30412605, 33.30412432, 33.30412256, 33.3041208, 33.30411902, 33.30411728, 33.30411554, 33.30411378, 33.30411208, 33.30411036, 33.30410866, 33.30410698, 33.30410535, 33.30410372, 33.30410208, 33.3041004, 33.30409893, 33.30409728, 33.30409564, 33.30409411, 33.30409238, 33.30409083, 33.30408919, 33.30408752, 33.30408579, 33.30408463, 33.30408295, 33.30408123, 33.30407952, 33.30407785, 33.30407608, 33.30407436, 33.30407267, 33.30407097, 33.30406947, 33.3040679, 33.3040663, 33.30406466, 33.30406313, 33.30406183, 33.30406054, 33.30405932, 33.30405816, 33.30405703, 33.30405602, 33.30405517, 33.30405467, 33.3040537, 33.3040528, 33.3040524, 33.30405185, 33.30405133, 33.30405083, 33.30405001, 33.30404917, 33.30404834, 33.30404755, 33.30404678, 33.30404617, 33.3040451, 33.30404427, 33.3040437, 33.30404327, 33.30404269, 33.3040423, 33.30404184, 33.304042, 33.30404195, 33.304042, 33.304042, 33.30404183, 33.30404183, 33.30404207, 33.30404239, 33.30404283, 33.30404317, 33.30404377, 33.30404442, 33.304045, 33.30404533, 33.30404583, 33.3040465, 33.30404726, 33.30404783, 33.30404846, 33.30404926, 33.30404999, 33.30405036, 33.30405112, 33.30405153, 33.30405183, 33.304052, 33.304052, 33.30405183, 33.30405167, 33.3040515, 33.30405117, 33.30405075, 33.30405026, 33.30404967, 33.30404883, 33.30404801, 33.30404694, 33.3040459, 33.30404467, 33.30404334, 33.30404195, 33.30404048, 33.30403893, 33.30403738, 33.30403588, 33.30403435, 33.30403281, 33.30403119, 33.30402962, 33.30402801, 33.30402632, 33.30402463, 33.30402292, 33.30402118, 33.30401944, 33.30401767, 33.3040159, 33.30401413, 33.30401239, 33.30401065, 33.30400895, 33.30400721, 33.30400546, 33.30400381, 33.3040023, 33.30400069, 33.30399913, 33.3039974, 33.30399581, 33.30399409, 33.3039925, 33.3039909, 33.30398913, 33.30398742, 33.30398599, 33.30398426, 33.30398249, 33.30398069, 33.30397899, 33.30397727, 33.30397559, 33.30397394, 33.30397251, 33.30397095, 33.30396971, 33.30396852, 33.30396728, 33.30396633, 33.30396522, 33.30396436, 33.30396343, 33.3039625, 33.30396166, 33.3039607, 33.30395983, 33.30395917, 33.30395857, 33.30395791, 33.30395748, 33.30395713, 33.30395691, 33.30395638, 33.30395615, 33.30395583, 33.30395537, 33.30395517, 33.303955, 33.30395479, 33.3039545, 33.3039545, 33.30395433, 33.30395449, 33.3039545, 33.30395467, 33.30395498, 33.30395517, 33.30395567, 33.303956, 33.3039565, 33.30395707, 33.30395764, 33.30395801, 33.30395885, 33.30395965, 33.3039606, 33.30396152, 33.30396255, 33.30396377, 33.30396516, 33.30396639, 33.30396774, 33.30396894, 33.3039701, 33.30397116, 33.30397211, 33.30397305, 33.3039739, 33.3039745, 33.30397529, 33.3039759, 33.30397652, 33.30397713, 33.30397757, 33.30397816, 33.30397867, 33.3039791, 33.30397968, 33.30398044, 33.30398105, 33.30398183, 33.30398257, 33.30398351, 33.30398444, 33.30398549, 33.30398658, 33.30398782, 33.30398919, 33.30399063, 33.30399212, 33.30399369, 33.30399528, 33.30399702, 33.3039987, 33.30400043, 33.30400218, 33.30400395, 33.3040057, 33.30400745, 33.30400925, 33.30401104, 33.30401281, 33.30401455, 33.30401628, 33.30401802, 33.30401979, 33.30402153, 33.30402328, 33.30402505, 33.30402683, 33.30402862, 33.30403041, 33.30403217, 33.30403395, 33.30403572, 33.30403748, 33.30403921, 33.30404092, 33.30404255, 33.30404408, 33.3040457, 33.30404725, 33.3040488, 33.30405033, 33.30405186, 33.30405334, 33.30405481, 33.30405638, 33.30405796, 33.30405946, 33.30406102, 33.30406263, 33.30406431, 33.30406604, 33.30406763, 33.30406942, 33.30407121, 33.30407296, 33.3040747, 33.3040764, 33.30407807, 33.3040797, 33.3040813, 33.3040829, 33.30408425, 33.30408563, 33.30408714, 33.30408845, 33.30408992, 33.30409134, 33.3040924, 33.30409342, 33.30409464, 33.30409566, 33.3040967, 33.30409745, 33.30409817, 33.30409869, 33.30409917, 33.30409917, 33.304099, 33.30409883, 33.30409867, 33.30409833, 33.304098, 33.3040975, 33.30409725, 33.3040969, 33.3040965, 33.30409617, 33.3040955, 33.304095, 33.30409449, 33.30409369, 33.30409306, 33.30409246, 33.30409169, 33.304091, 33.30409039, 33.30408964, 33.30408894, 33.3040879, 33.30408698, 33.30408609, 33.30408501, 33.30408417, 33.30408299, 33.30408207, 33.30408113, 33.30408011, 33.30407914, 33.30407806, 33.30407703, 33.30407611, 33.30407529, 33.30407472, 33.30407402, 33.30407336, 33.30407299, 33.3040725, 33.30407233, 33.30407238, 33.30407254, 33.30407298, 33.30407362, 33.30407437, 33.30407524, 33.30407621, 33.30407732, 33.30407842, 33.30407964, 33.30408083, 33.30408199, 33.30408313, 33.30408433, 33.30408554, 33.30408674, 33.30408795, 33.30408915, 33.30409035, 33.30409162, 33.30409282, 33.30409406, 33.3040955, 33.30409691, 33.30409843, 33.30409996, 33.30410145, 33.30410302, 33.30410462, 33.30410625, 33.30410785, 33.30410955, 33.30411127, 33.30411299, 33.30411473, 33.3041165, 33.30411826, 33.30412002, 33.3041218, 33.30412359, 33.30412539, 33.30412719, 33.30412898, 33.30413077, 33.30413253, 33.30413431, 33.30413605, 33.30413782, 33.30413955, 33.30414131, 33.30414306, 33.30414477, 33.30414638, 33.30414793, 33.30414969, 33.30415133, 33.3041531, 33.30415478, 33.30415644, 33.30415803, 33.30415973, 33.30416129, 33.30416291, 33.30416462, 33.30416633, 33.304168, 33.30416971, 33.30417146, 33.30417317, 33.30417477, 33.30417655, 33.3041779, 33.30417967, 33.30418145, 33.30418304, 33.3041847, 33.30418622, 33.30418767, 33.30418921, 33.30419068, 33.30419227, 33.3041935, 33.30419503, 33.30419648, 33.30419779, 33.30419913, 33.30420041, 33.30420146, 33.3042027, 33.30420372, 33.30420454, 33.30420533, 33.30420584, 33.30420642, 33.30420683, 33.30420714, 33.30420733, 33.3042075, 33.30420766, 33.30420718, 33.30420712, 33.30420667, 33.30420623, 33.30420586, 33.3042055, 33.30420497, 33.30420459, 33.30420417, 33.30420367, 33.30420313, 33.30420267, 33.30420217, 33.30420167, 33.30420133, 33.30420076, 33.30420033, 33.30419983, 33.30419933, 33.30419882, 33.30419833, 33.30419768, 33.30419719, 33.30419672, 33.30419617, 33.30419572, 33.30419522, 33.3041945, 33.30419416, 33.30419352, 33.304193, 33.30419279, 33.3041925, 33.30419233, 33.30419233, 33.30419233, 33.30419253, 33.30419283, 33.30419322, 33.30419371, 33.30419407, 33.30419475, 33.30419544, 33.30419625, 33.30419702, 33.30419805, 33.30419893, 33.30419998, 33.30420102, 33.30420207, 33.30420327, 33.30420455, 33.30420578, 33.30420717, 33.30420853, 33.3042099, 33.30421136, 33.30421282, 33.30421437, 33.3042159, 33.30421751, 33.30421912, 33.30422079, 33.30422245, 33.30422418, 33.30422586, 33.30422757, 33.30422929, 33.30423105, 33.30423274, 33.30423443, 33.30423617, 33.3042379, 33.30423964, 33.30424139, 33.30424306, 33.30424479, 33.30424652, 33.304248, 33.30424976, 33.30425154, 33.3042533, 33.30425509, 33.30425689, 33.30425867, 33.30426047, 33.30426226, 33.30426403, 33.30426571, 33.30426735, 33.30426908, 33.30427076, 33.30427248, 33.30427415, 33.30427584, 33.30427738, 33.30427906, 33.30428065, 33.30428205, 33.3042837, 33.30428506, 33.30428645, 33.304288, 33.30428946, 33.30429098, 33.3042922, 33.3042936, 33.30429462, 33.30429558, 33.30429638, 33.304297, 33.30429767, 33.30429832, 33.30429893, 33.30429939, 33.30429967, 33.30429983, 33.30429985, 33.30429968, 33.30429967, 33.3042996, 33.3042994, 33.3042995, 33.30429933, 33.30429917, 33.30429894, 33.30429855, 33.30429831, 33.30429783, 33.30429737, 33.30429697, 33.3042965, 33.30429608, 33.3042955, 33.30429506, 33.3042946, 33.30429398, 33.30429343, 33.30429291, 33.30429233, 33.304292, 33.30429138, 33.304291, 33.30429068, 33.30429037, 33.30428989, 33.30428967, 33.3042895, 33.3042895, 33.3042894, 33.30428929, 33.30428919, 33.3042903, 33.30429148, 33.30429252, 33.30429368, 33.30429483, 33.30429598, 33.30429714, 33.30429826, 33.30429944, 33.30430063, 33.30430181, 33.30430287, 33.30430407, 33.3043052, 33.30430642, 33.30430753, 33.30430867, 33.30430985, 33.30431089, 33.3043121, 33.30431337, 33.30431456, 33.30431579, 33.30431698, 33.30431833, 33.30431958, 33.30432092, 33.30432214, 33.30432347, 33.30432474, 33.30432609, 33.30432748, 33.30432867, 33.30433003, 33.30433133, 33.30433263, 33.30433399, 33.30433523, 33.30433657, 33.30433797, 33.30433937, 33.30434067, 33.304342, 33.30434334, 33.30434457, 33.30434591, 33.30434725, 33.30434867, 33.30434997, 33.30435138, 33.30435259, 33.30435392, 33.3043552, 33.30435656, 33.3043579, 33.30435921, 33.3043605, 33.30436182, 33.3043631, 33.30436435, 33.30436565, 33.30436696, 33.30436823, 33.30436946, 33.30437072, 33.30437193, 33.30437319, 33.30437442, 33.30437563, 33.30437672, 33.30437784, 33.30437898, 33.30438002, 33.30438112, 33.3043822, 33.30438318, 33.30438427, 33.30438535, 33.30438643, 33.30438748, 33.30438854, 33.30438969, 33.30439078, 33.30439199, 33.30439309, 33.30439426, 33.30439549, 33.3043967, 33.30439793, 33.30439917, 33.30440042, 33.30440174, 33.30440304, 33.30440434, 33.30440563, 33.30440699, 33.30440833, 33.30440962, 33.30441093, 33.30441225, 33.30441349, 33.30441479, 33.30441613, 33.30441739, 33.30441862, 33.30441985, 33.3044211, 33.30442234, 33.30442362, 33.30442493, 33.3044262, 33.30442739, 33.30442869, 33.30442987, 33.30443116, 33.30443233, 33.30443357, 33.30443475, 33.30443596, 33.30443707, 33.30443833, 33.30443962, 33.30444082, 33.30444186, 33.30444294]
  in  "HENES":refnum<visa-resource-name>="COM3"
  out "E-STOP":bool
  out "Remote_M/A":bool
  out "Steer_Feed":dbl
  out "Alive_PCU":u8(slide) scale=0.0..254.0
  out "Gear_Feed":u8
  out "Speed_Feed(RPM)":dbl format="%#_g rpm"
  out "버퍼 읽기":string
  out "Speed_Feed(m/s)":dbl
  in  "HLV_Gear":u8
  in  "HLV_A/M":bool=TRUE
  in  "HLV_E-stop":bool
  out "버퍼 쓰기":string
  in  "InputSpeed":i16
  out "HENES Loop Time":u32=20
  in  "Steer Selector":enum32{"Stanley Method", "Pure Pursuit"}(radio)
  in  "Ld(m)":dbl=5.0 format="%#_13g"
  out "GPS":T1(graph)=[{"y_long_path"=[250243.79385612707], "x_lat_path"=[3688223.5281783747]}, {"y_long_path"=[250243.757], "x_lat_path"=[3688223.39]}, {"y_long_path"=array[944 elements], "x_lat_path"=array[944 elements]}, {"y_long_path"=[250246.8301, 250246.6716, 250246.4873, 250246.296, 250246.122, 250245.9257, 250245.7732, 250245.5875, 250245.3989, 250245.2166, 250245.0276, 250244.8653, 250244.6749, 250244.5098, 250244.319, 250244.1293, 250243.9404, 250243.757, 250243.5653, 250243.3909, 250243.2171, 250243.0265, 250242.8469, 250242.6561, 250242.4779, 250242.2931, 250242.1112, 250241.9363, 250241.7611, 250241.5908], "x_lat_path"=[3688223.612, 3688223.681, 3688223.731, 3688223.77, 3688223.796, 3688223.82, 3688223.842, 3688223.793, 3688223.791, 3688223.745, 3688223.702, 3688223.665, 3688223.63, 3688223.575, 3688223.538, 3688223.496, 3688223.445, 3688223.39, 3688223.345, 3688223.293, 3688223.242, 3688223.21, 3688223.151, 3688223.108, 3688223.058, 3688223.007, 3688222.954, 3688222.905, 3688222.836, 3688222.787]}]
  out "Tracking_Err(m)":dbl=4862130.802033398
  out "GPS_Steer_CMD(Deg)":dbl=2.9943056426975447
  in  "Input_Spd(kph)":dbl
  out "RDDF_Velocity":dbl=126.317125
  out "Output_Spd_CMD(%)":dbl
  out "WP_no.":i32=675
  in  "Map Refresh":bool
  in  "RDDF":path=path "C:/Users/JungiHong/OneDrive/Hongik/HI-RACE/2026-01/ExperimentModules/GPSPathTracking/1_5_map/1_5_map hard.txt"
  in  "k(Gain)":dbl=1.0 format="%#_13g"
  out "yi":dbl=3688223.293
  out "xi":dbl=250243.3909
  out "CTE":dbl=-0.11220359033506931
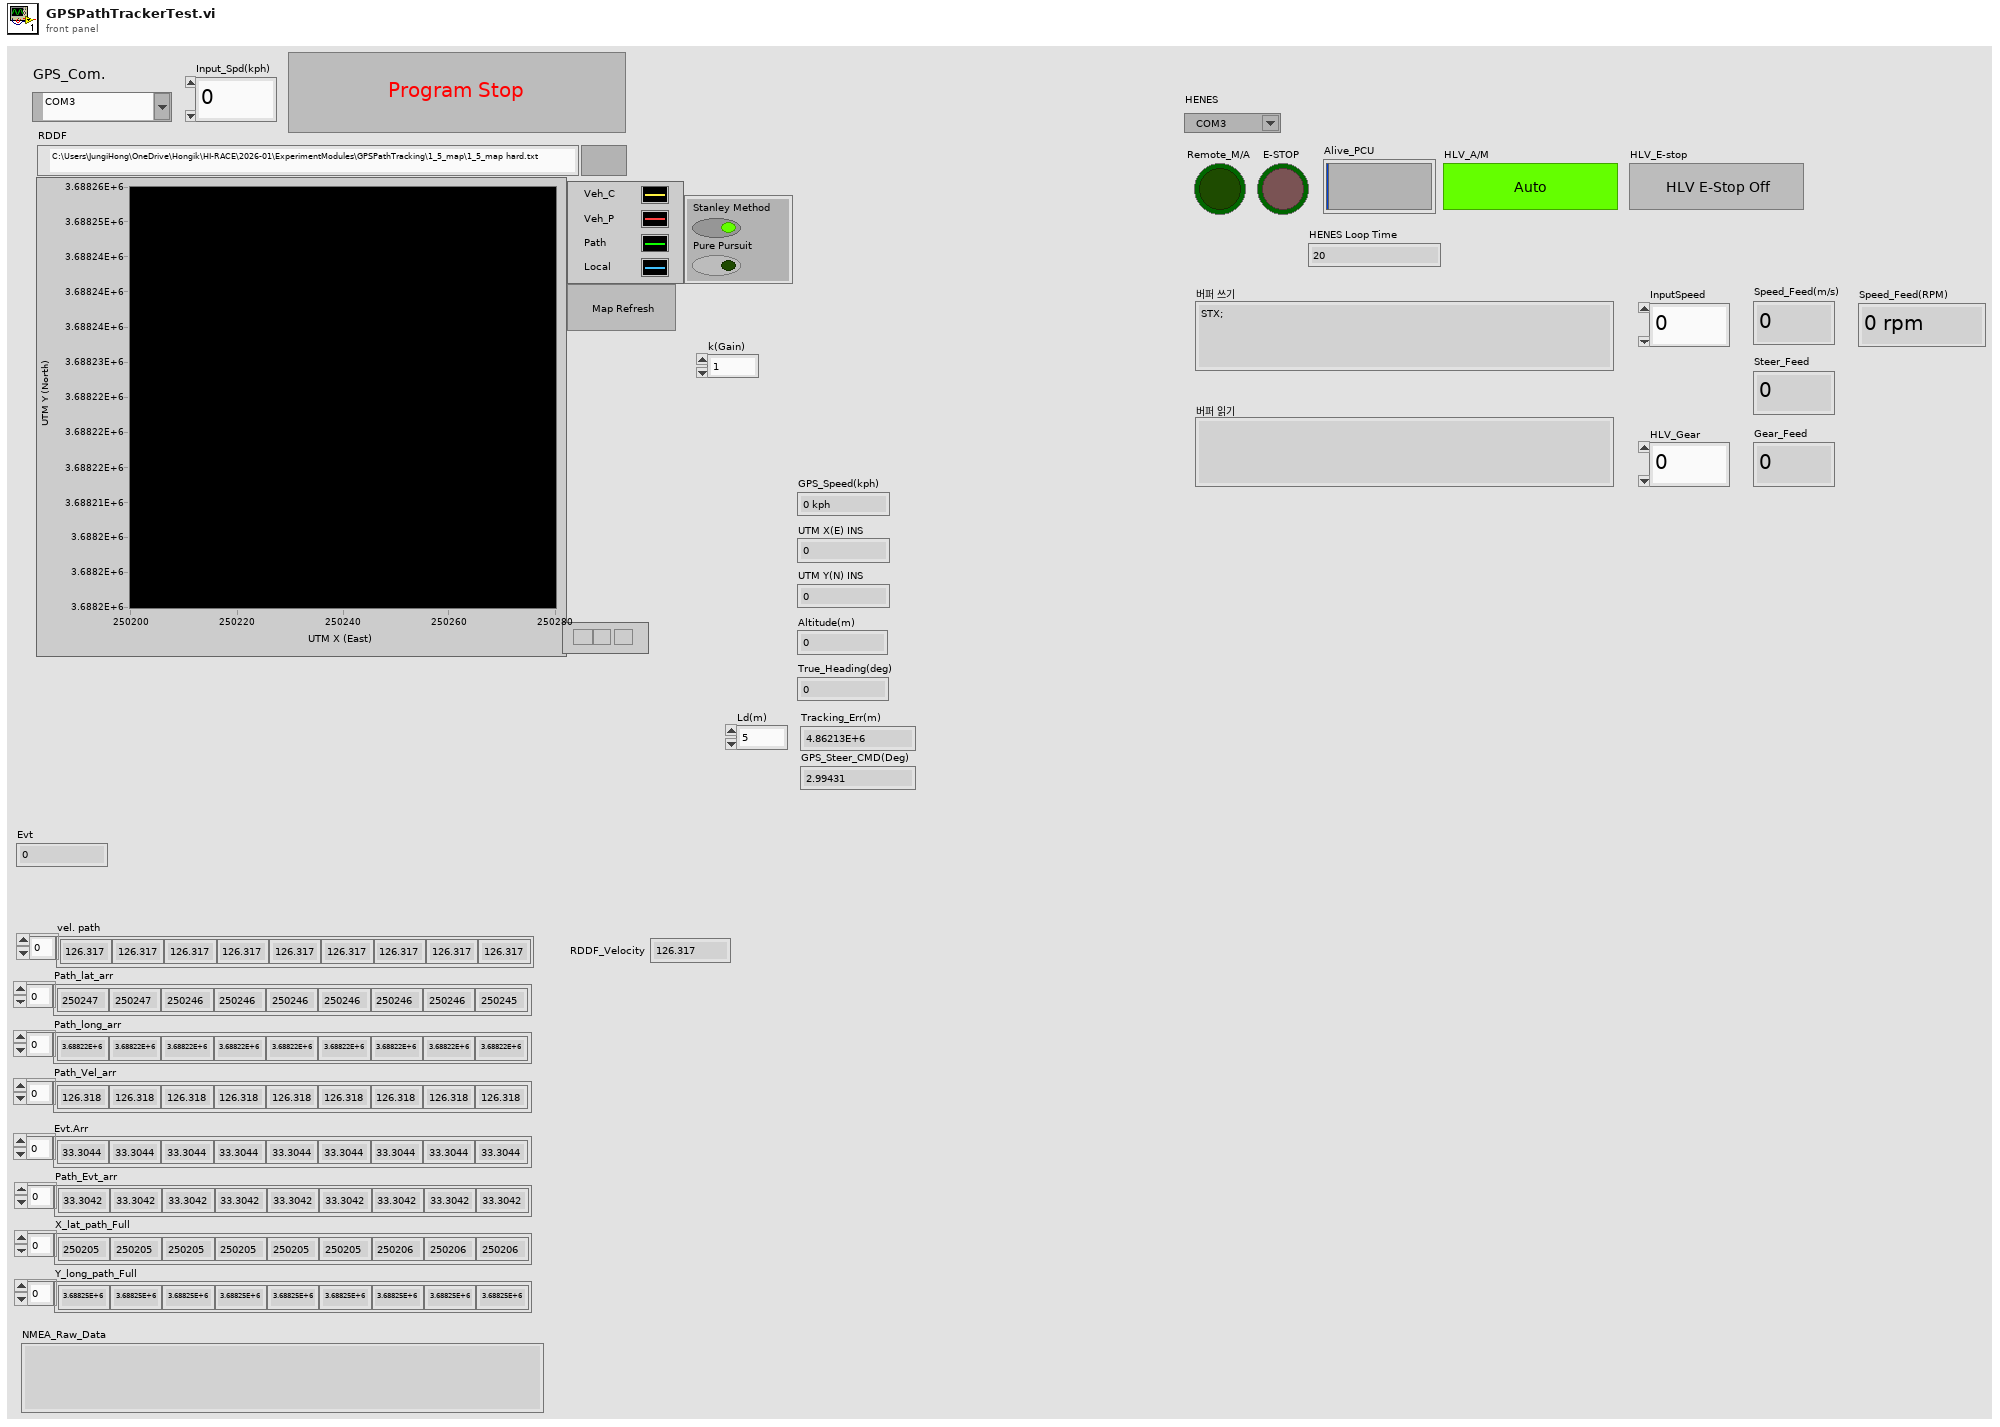
[diagram p1: front panel]
types:
  T1 = cluster{"y_long_path":dbl[], "x_lat_path":dbl[]}[]
  T2 = cluster{"HENES_M/A":u8, "HENES_E-Stop":u8, "HENES_Gear":u8, "HENES_Speed":i16, "HENES_Steer":i16, "HENES_Alive":u8}
  T3 = typedef "VISA Flush IO Buffer Mask.ctl" = u16
  T4 = typedef "VISA Set IO Buffer Mask.ctl" = u16
  T5 = cluster{"HLV_M/A_Status":u8, "HLV_E-Stop":u8, "HLV_Gear":u8, "HLV_Speed":i16, "HLV_Steer":i16, "HLV_Alive":u8}
  T6 = cluster{"oldest read timestamp":dbl, "latitude (deg)":dbl, "longitude (deg)":dbl, "ground speed (kph)":dbl, "true track angle (deg)":dbl, "altitude above mean sea level (m)":dbl}
  T7 = cluster{"X_lat_path_Full":dbl[], "Y_long_path_Full":dbl[]}
  T8 = cluster{"Path_lat_arr":dbl[], "Path_long_arr":dbl[]}
  T9 = cluster{"Path_lat_arr":dbl[], "Path_long_arr":dbl[]}[]
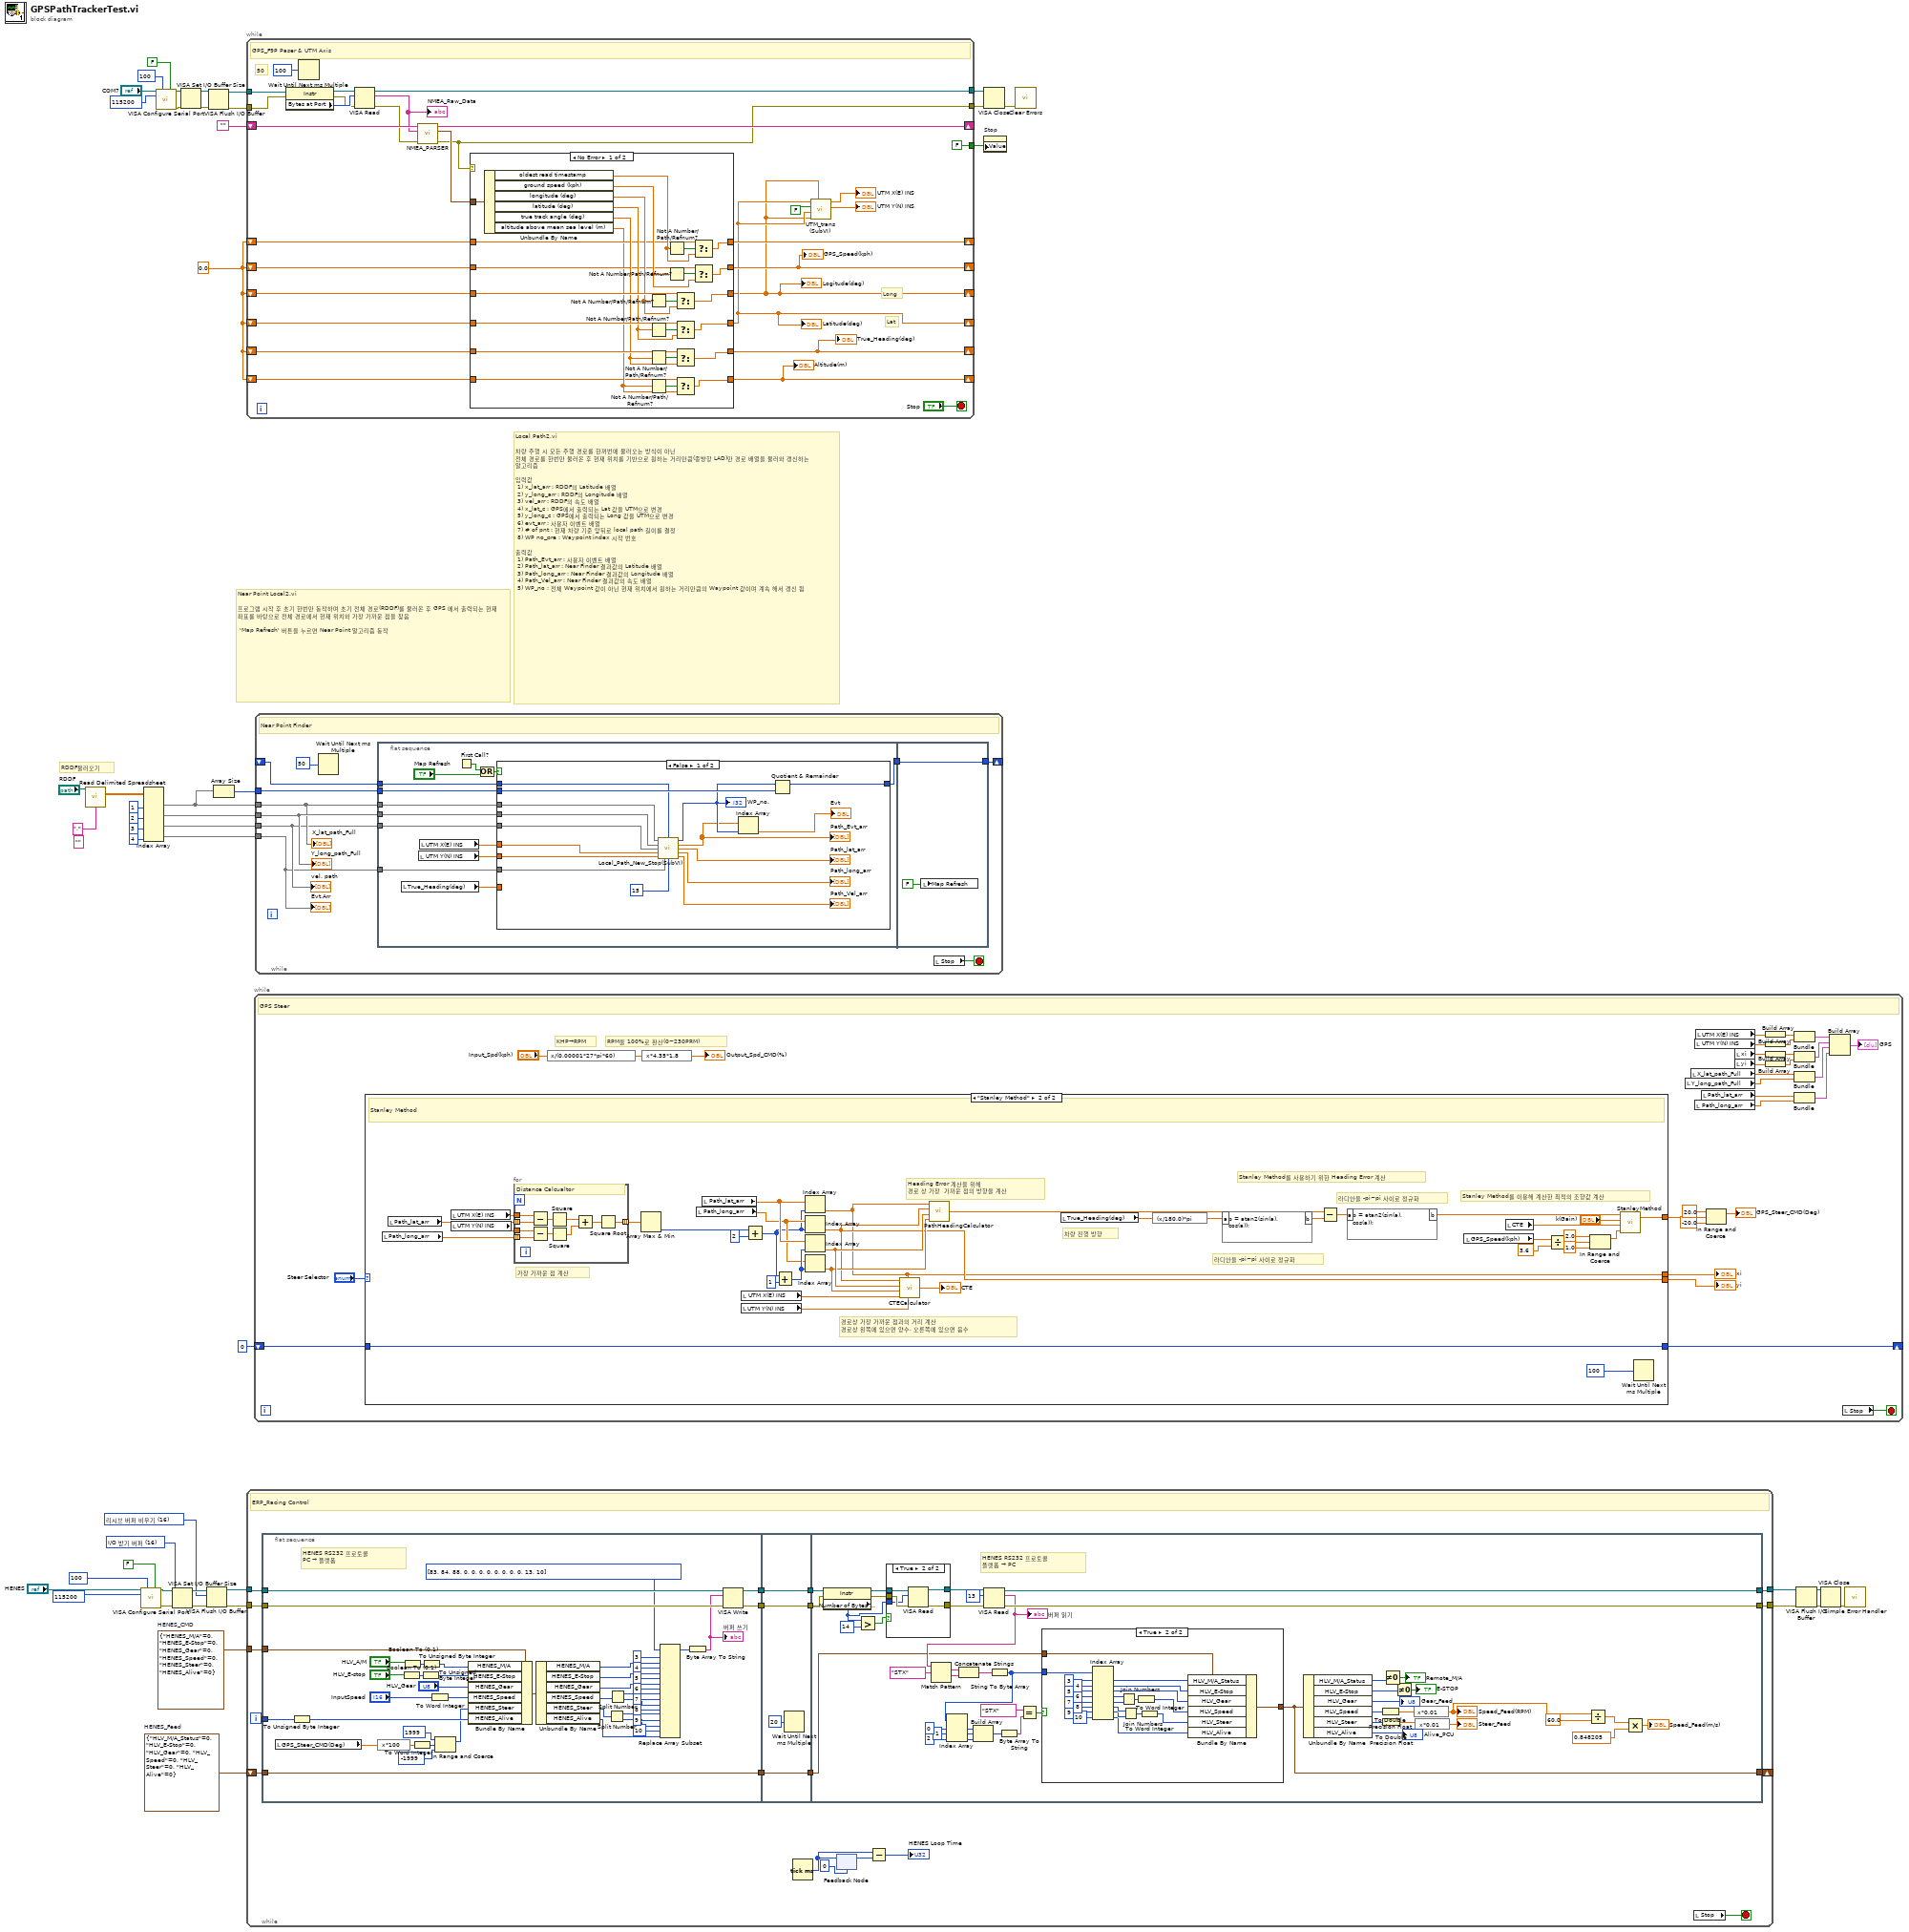
[diagram p0: block diagram]
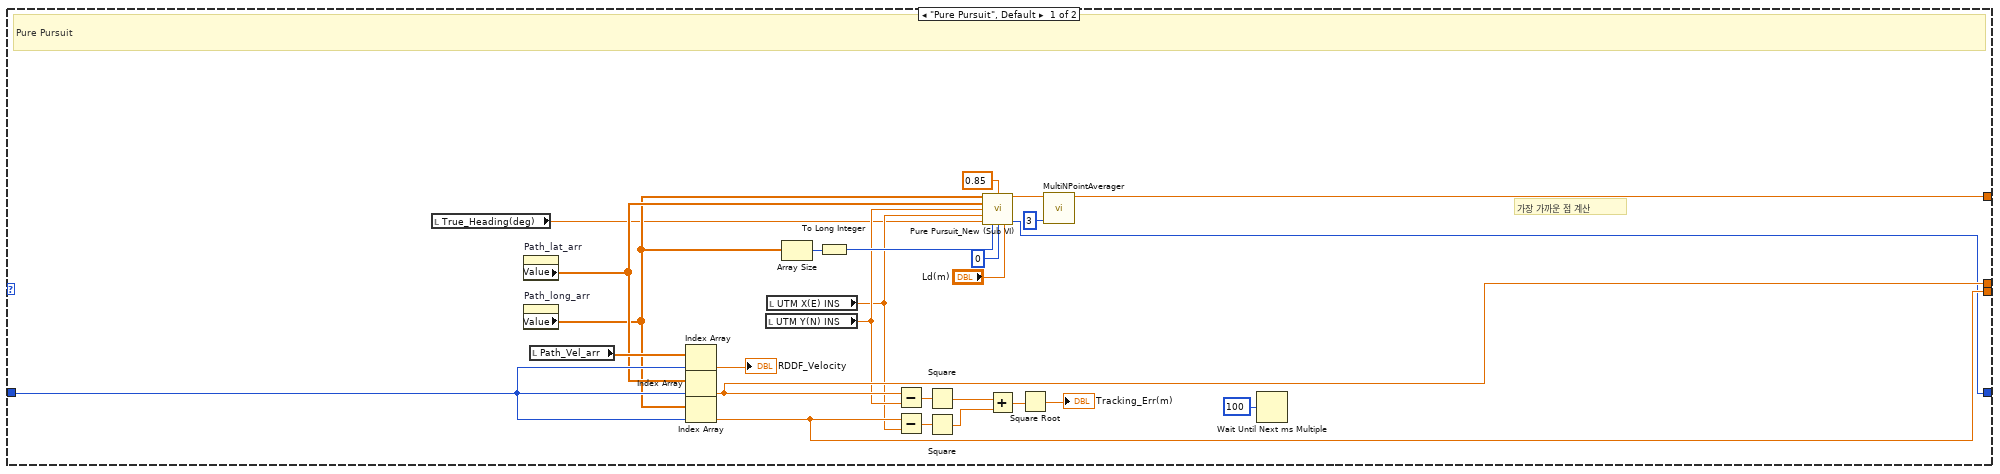
[diagram p5: hidden frame]
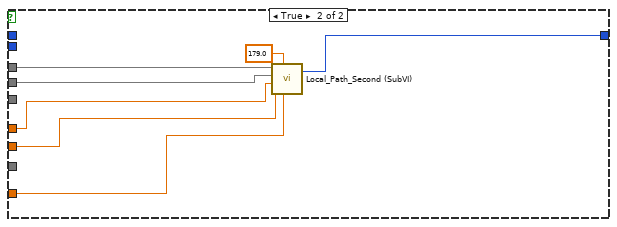
[diagram p6: hidden frame]
diagram:
  w16 = 0.0 ("x")
  w19 = T2 {"HENES_M/A"=0, "HENES_E-Stop"=0, "HENES_Gear"=0, "HENES_Speed"=0, "HENES_Steer"=0, "HENES_Alive"=0}  # HENES_CMD
  w22 = T3 16 items=["리시브 버퍼 비우기"=16, "전달 버퍼 디바이스에 쓰기"=32, "리시브 버퍼 비우기(I/O 없음)"=64, "전달 버퍼 비우기"=128] ("Mask")
  w25 = T4 16 items=["I/O 받기 버퍼"=16, "I/O 전달 버퍼"=32, "I/O 받기와 전달 버퍼"=48] ("Mask")
  w29 = T5 {"HLV_M/A_Status"=0, "HLV_E-Stop"=0, "HLV_Gear"=0, "HLV_Speed"=0, "HLV_Steer"=0, "HLV_Alive"=0}  # HENES_Feed
  (unwired) "" ("delimiter (\\t)")
  # "Near Point Local2.vi\n\n프로그램 시작 후 초기 한번만 동작하며 초기 전체 경로(RDDF)를 불러온 후 GPS 에서 출력되는 현재 좌표를 바탕으로 전체 경로에서 현재 위치와 가장 가까운 점을 찾음\n\n 'Map Refresh' 버튼을 누르면 Near Point 알고리즘 동작"
  # "Local Path2.vi\n\n차량 주행 시 모든 주행 경로를 한꺼번에 불러오는 방식이 아닌\n전체 경로를 한번만 불러온 후 현재 위치를 기반으로 원하는 거리만큼(종뱡항 LAD)만 경로 배열을 불러와 갱신하는 알고리즘\n\n입력값 \n 1) x_lat_arr : RDDF의 Latitude 배열\n 2) y_long_arr : RDDF의 Longitude 배열\n 3) vel_arr : RDDF의 속도 배열\n 4) x_lat_c : GPS에서 출력되는 Lat 값을 UTM으로 변경\n 5) y_long_c : GPS에서 출력되는 Long 값을 UTM으로 변경\n 6) evt_arr : 사용자 이벤트 배열\n 7) # of pnt : 현재 차량 기준 앞뒤로 local path 길이를 결정\n 8) WP no_pre : Waypoint index 시작 번호\n\n출력값 \n 1) Path_Evt_arr : 사용자 이벤트 배열\n 2) Path_lat_arr : Near Finder 결과값의 Latitude 배열\n 3) Path_long_arr : Near Finder 결과값의 Longitude 배열\n 4) Path_Vel_arr : Near Finder 결과값의 속도 배열\n 5) WP_no : 전체 Waypoint 값이 아닌 현재 위치에서 원하는 거리만큼의 Waypoint 값이며 계속 해서 갱신 됨"
  # "RDDF불러오기"
  n1 = call-poly <vilib>:"Read Delimited Spreadsheet.vi"("file path (dialog if empty)"="RDDF", "delimiter (\\t)"="," ("delimiter (\\t)")) -> ("all rows"=w43:dbl[][])  [unwired: 8 in, 5 out]
  n2 = call-poly "VISA Configure Serial Port"("VISA resource name"="HENES", "timeout (10sec)"=u32 100, "Enable Termination\nChar (T)"=FALSE ("Enable Termination\nChar (T)"), "baud rate (9600)"=u32 115200) -> ("VISA resource name out"=w21:refnum<visa-resource-name>, "error out"=w20:errorcluster)  [unwired: 10 in]
  n3 = Index Array(array=w43, index (col) #1=1 ("비활성화된 인덱스 (열)"), index (col) #2=2 ("인덱스 (열)"), index (col) #3=3 ("인덱스 (열)"), index (col) #4=4 ("인덱스 (열)")) -> (element #1=w41:dbl[], element #2=w40:dbl[], element #3=w38:dbl[], element #4=w39:dbl[])  [unwired: 4 in]
  n4 = call-poly "VISA Configure Serial Port"("VISA resource name"="COM7", "timeout (10sec)"=u32 100, "Enable Termination\nChar (T)"=FALSE ("Enable Termination\nChar (T)"), "baud rate (9600)"=u32 115200) -> ("VISA resource name out"=w10:refnum<visa-resource-name>, "error out"=w11:errorcluster)  [unwired: 10 in]
  n5 = VISA Set I/O Buffer Size(VISA resource name=w21, mask (16)=w25, error in (no error)=w20) -> (VISA resource name out=w24:refnum<visa-resource-name>, error out=w23:errorcluster)  [unwired: 1 in]
  n6 = VISA Set I/O Buffer Size(VISA resource name=w10, error in (no error)=w11) -> (VISA resource name out=w4:refnum<visa-resource-name>, error out=w5:errorcluster)  [unwired: 2 in]
  n7 = VISA Flush I/O Buffer(VISA resource name=w24, mask (16)=w22, error in (no error)=w23) -> (VISA resource name out=w34:refnum<visa-resource-name>, error out=w33:errorcluster)
  n8 = VISA Flush I/O Buffer(VISA resource name=w4, error in (no error)=w5) -> (VISA resource name out=w6:refnum<visa-resource-name>, error out=w7:errorcluster)  [unwired: 1 in]
  n9 = Array Size(array=w41) -> (size(s)=w42:i32)
  n10 = while {
    tunnel: w6 -> [w76]
    tunnel: w7 -> [w74]
    tunnel: [w78] -> w1
    tunnel: [w66] -> w3
    shift-right: [w67] -> _
    shift-left: "" -> [w71]
    shift-right: [w53] -> _
    shift-left: w16 -> [w65]
    shift-right: [w51] -> _
    shift-left: w16 -> [w64]
    shift-right: [w52] -> _
    shift-left: w16 -> [w63]
    shift-right: [w59] -> _
    shift-left: w16 -> [w62]
    shift-right: [w58] -> _
    shift-left: w16 -> [w61]
    tunnel: [FALSE] -> w9
    shift-right: [w49] -> _
    shift-left: w16 -> [w50]
    stop <- "Stop" stop-if-true
    # "Lat"
    # "Long"
    # "50"
    # "GPS_F9P Paser & UTM Axis"
    n11 = property class="Instr"(reference=w76, error in=w74) -> (reference out=w75:refnum<visa-resource-name>, error out=w73:errorcluster, "Bytes at Port"=w77:u32)
    n12 = Wait Until Next ms Multiple(millisecond multiple=u32 100) -> ()  [unwired: 1 out]
    n13 = VISA Read(VISA resource name=w75, byte count=w77, error in (no error)=w73) -> (VISA resource name out=w78:refnum<visa-resource-name>, read buffer=w70:string, error out=w68:errorcluster)  [unwired: 1 out]
    "NMEA_Raw_Data" <- w70
    n14 = call "NMEA_PARSER.vi"("previous partial sentence"=w71, "sensor data"=w70, "error in (no error)"=w68) -> ("remaining partial sentence"=w67:string, "GPS data"=w69:T6, "error out"=w66:errorcluster)  [unwired: 5 in]
    n15 = case shown="No Error" w66 {
      tunnel: w69 -> [w103 _]
      tunnel: w64 -> [w99 w109]
      tunnel: w63 -> [w98 w108]
      tunnel: w62 -> [w97 w107]
      tunnel: [w93 w109] -> w51
      tunnel: [w92 w108] -> w52
      tunnel: [w91 w107] -> w59
      tunnel: w65 -> [w88 w106]
      tunnel: [w87 w106] -> w53
      tunnel: w61 -> [w84 w105]
      tunnel: [w83 w105] -> w58
      tunnel: [w80 w104] -> w49
      tunnel: w50 -> [w79 w104]
      frame No Error {
        n16 = Unbundle By Name(w103) -> ("oldest read timestamp"=w85:dbl, "ground speed (kph)"=w89:dbl, "longitude (deg)"=w96:dbl, "latitude (deg)"=w95:dbl, "true track angle (deg)"=w94:dbl, "altitude above mean sea level (m)"=w81:dbl)
        n17 = Not A Number/Path/Refnum?(number/path/refnum=w96) -> (NaN/Path/Refnum?=w102:bool)
        n18 = Not A Number/Path/Refnum?(number/path/refnum=w95) -> (NaN/Path/Refnum?=w101:bool)
        n19 = Not A Number/Path/Refnum?(number/path/refnum=w94) -> (NaN/Path/Refnum?=w100:bool)
        n20 = Not A Number/Path/Refnum?(number/path/refnum=w81) -> (NaN/Path/Refnum?=w82:bool)
        n21 = Not A Number/Path/Refnum?(number/path/refnum=w85) -> (NaN/Path/Refnum?=w86:bool)
        n22 = Not A Number/Path/Refnum?(number/path/refnum=w89) -> (NaN/Path/Refnum?=w90:bool)
        n23 = Select(t=w99, s=w102, f=w96) -> (s? t:f=w93:dbl)
        n24 = Select(t=w98, s=w101, f=w95) -> (s? t:f=w92:dbl)
        n25 = Select(t=w97, s=w100, f=w94) -> (s? t:f=w91:dbl)
        n26 = Select(t=w79, s=w82, f=w81) -> (s? t:f=w80:dbl)
        n27 = Select(t=w84, s=w86, f=w85) -> (s? t:f=w83:dbl)
        n28 = Select(t=w88, s=w90, f=w89) -> (s? t:f=w87:dbl)
      }
      frame Error {
        # "Invalid data points."
      }
    }
    "True_Heading(deg)" <- w59
    "GPS_Speed(kph)" <- w53
    "Latitude(deg)" <- w52
    "Logitude(deg)" <- w51
    "Altitude(m)" <- w49
    n29 = call "UTM_trans (SubVI).vi"("Long_Deg"=w51, "long"=w51, "lat"=w52, "East?West?"=FALSE, "Lat_Deg"=w52) -> ("UTM_Y(Northing)"=→"UTM Y(N) INS":dbl, "UTM_X(Easting)"=→"UTM X(E) INS":dbl)  [unwired: 2 out]
  }
  n30 = while {
    tunnel: w34 -> [w128]
    tunnel: w33 -> [w127]
    tunnel: [w121] -> w32
    tunnel: [w120] -> w31
    shift-right: [w115] -> _
    shift-left: w29 -> [w118]
    tunnel: w19 -> [w116]
    i -> [w122]
    stop <- w110 stop-if-true
    # "ERP_Racing Control"
    n31 = flat-sequence {
      tunnel: [w171] -> w125
      tunnel: [w170] -> w123
      tunnel: w128 -> [w173]
      tunnel: w127 -> [w172]
      tunnel: w122 -> [w169]
      tunnel: [w168] -> w119
      tunnel: w118 -> [w168]
      tunnel: w116 -> [w167]
      tunnel: [w177] -> w126
      tunnel: w125 -> [w177]
      tunnel: [w176] -> w124
      tunnel: w123 -> [w176]
      tunnel: w119 -> [w174]
      tunnel: [w174] -> w117
      tunnel: w126 -> [w205]
      tunnel: w124 -> [w204]
      tunnel: [w222] -> w121
      tunnel: [w221] -> w120
      tunnel: w117 -> [w196]
      tunnel: [w194] -> w115
      frame #0 {
        # "HENES RS232 프로토콜\nPC → 플랫폼"
        n32 = local read "GPS_Steer_CMD(Deg)"() -> (w129:dbl)
        n33 = To Unsigned Byte Integer(number=w169) -> (unsigned 8bit integer=w158:u8)
        n34 = expression code="x*100"(w129) -> (w133:dbl)
        n35 = Boolean To (0,1)(Boolean="HLV_E-stop") -> (0, 1=w153:i16)
        n36 = Boolean To (0,1)(Boolean="HLV_A/M") -> (0, 1=w154:i16)
        n37 = To Word Integer(number=w133) -> (16bit integer=w136:i16)
        n38 = To Unsigned Byte Integer(number=w153) -> (unsigned 8bit integer=w151:u8)
        n39 = To Unsigned Byte Integer(number=w154) -> (unsigned 8bit integer=w152:u8)
        n40 = To Word Integer(number="InputSpeed") -> (16bit integer=w145:i16)
        n41 = In Range and Coerce(upper limit=i16 1999 ("상위 리미트"), x=w136, lower limit=i16 -1999 ("상위 리미트")) -> (coerced(x)=w144:i16)  [unwired: 1 out]
        n42 = Bundle By Name(cluster=w167, "HENES_M/A"=w152, "HENES_E-Stop"=w151, "HENES_Gear"="HLV_Gear", "HENES_Speed"=w145, "HENES_Steer"=w144, "HENES_Alive"=w158) -> (w160:T2)
        n43 = Unbundle By Name(w160) -> ("HENES_M/A"=w148:u8, "HENES_E-Stop"=w147:u8, "HENES_Gear"=w137:u8, "HENES_Speed"=w140:i16, "HENES_Steer"=w143:i16, "HENES_Alive"=w157:u8)
        n44 = Split Number(x=w143) -> (hi(x)=w142:u8, lo(x)=w141:u8)
        n45 = Split Number(x=w140) -> (hi(x)=w139:u8, lo(x)=w138:u8)
        n46 = Replace Array Subset(array=u8[] [83, 84, 88, 0, 0, 0, 0, 0, 0, 0, 0, 13, 10] ("unsigned byte array"), new element #1=w148, index #1=3, new element #2=w147, index #2=4, new element #3=w137, index #3=5, new element #4=w139, index #4=6, new element #5=w138, index #5=7, new element #6=w142, index #6=8, new element #7=w141, index #7=9, new element #8=w157, index #8=10) -> (w130:u8[])
        n47 = Byte Array To String(unsigned byte array=w130) -> (string=w132:string)
        "버퍼 쓰기" <- w132
        n48 = VISA Write(VISA resource name=w173, write buffer=w132, error in (no error)=w172) -> (VISA resource name out=w171:refnum<visa-resource-name>, error out=w170:errorcluster)  [unwired: 1 out]
      }
      frame #1 {
        n49 = Wait Until Next ms Multiple(millisecond multiple=u32 20 ("대기 시간 (ms)")) -> ()  [unwired: 1 out]
      }
      frame #2 {
        # "HENES RS232 프로토콜\n플랫폼 → PC"
        n50 = property class="Instr"(reference=w205, error in=w204) -> (reference out=w185:refnum<visa-resource-name>, error out=w184:errorcluster, "Serial Settings:Number of Bytes at Serial Port"=w183:u32)
        n51 = Greater?(x=w183, y=u32 14) -> (0:w201:bool)
        n52 = case shown="True" w201 {
          tunnel: w185 -> [w249 w254]
          tunnel: w184 -> [w248 w253]
          tunnel: [w249 w252] -> w203
          tunnel: [w248 w251] -> w202
          tunnel: w183 -> [_ w250]
          frame False {
          }
          frame True {
            n53 = VISA Read(VISA resource name=w254, byte count=w250, error in (no error)=w253) -> (VISA resource name out=w252:refnum<visa-resource-name>, error out=w251:errorcluster)  [unwired: 2 out]
          }
        }
        n54 = VISA Read(VISA resource name=w203, byte count=u32 13, error in (no error)=w202) -> (VISA resource name out=w222:refnum<visa-resource-name>, read buffer=w220:string, error out=w221:errorcluster)  [unwired: 1 out]
        "버퍼 읽기" <- w220
        n55 = Match Pattern(string=w220, regular expression="STX") -> (match substring=w217:string, after substring=w218:string)  [unwired: 1 in, 2 out]
        n56 = Concatenate Strings(w217, w218) -> (w216:string)
        n57 = String To Byte Array(string=w216) -> (unsigned byte array=w198:u8[])
        n58 = Index Array(array=w198, index #1=0, index #2=1, index #3=2) -> (element #1=w211:u8, element #2=w210:u8, element #3=w209:u8)
        n59 = Build Array(w211, w210, w209) -> (w208:u8[])
        n60 = Byte Array To String(unsigned byte array=w208) -> (string=w206:string)
        n61 = Equal?(x="STX", y=w206) -> (x = y?=w197:bool)
        n62 = case shown="True" w197 {
          tunnel: w198 -> [_ w247]
          tunnel: [w224 w234] -> w194
          tunnel: w196 -> [w224 w236]
          frame False {
          }
          frame True {
            n63 = Index Array(array=w247, index #1=3, index #2=4, index #3=5, index #4=6, index #5=7, index #6=8, index #7=9, index #8=10) -> (element #1=w235:u8, element #2=w233:u8, element #3=w232:u8, element #4=w231:u8, element #5=w230:u8, element #6=w228:u8, element #7=w227:u8, element #8=w225:u8)
            n64 = Join Numbers(hi=w231, lo=w230) -> ((hi.lo)=w238:u16)
            n65 = Join Numbers(hi=w228, lo=w227) -> ((hi.lo)=w237:u16)
            n66 = To Word Integer(number=w238) -> (16bit integer=w229:i16)
            n67 = To Word Integer(number=w237) -> (16bit integer=w226:i16)
            n68 = Bundle By Name(cluster=w236, "HLV_M/A_Status"=w235, "HLV_E-Stop"=w233, "HLV_Gear"=w232, "HLV_Speed"=w229, "HLV_Steer"=w226, "HLV_Alive"=w225) -> (w234:T5)
          }
        }
        n69 = Unbundle By Name(w194) -> ("HLV_M/A_Status"=w195:u8, "HLV_E-Stop"=w189:u8, "HLV_Gear"=→"Gear_Feed":u8, "HLV_Speed"=w187:i16, "HLV_Steer"=w186:i16, "HLV_Alive"=→"Alive_PCU":u8)
        n70 = To Double Precision Float(number=w187) -> (double precision float=w199:dbl)
        n71 = To Double Precision Float(number=w186) -> (double precision float=w192:dbl)
        n72 = Not Equal To 0?(x=w195) -> (x != 0?=→"Remote_M/A":bool)
        n73 = Not Equal To 0?(x=w189) -> (x != 0?=→"E-STOP":bool)
        n74 = expression code="x*0.01"(w199) -> (w178:dbl)
        "Speed_Feed(RPM)" <- w178
        n75 = expression code="x*0.01"(w192) -> (→"Steer_Feed":dbl)
        n76 = Divide(x=w178, y=60.0) -> (x/y=w182:dbl)
        n77 = Multiply(x=w182, y=0.848205) -> (x*y=→"Speed_Feed(m/s)":dbl)
      }
    }
    n78 = Tick Count (ms)() -> (millisecond timer value=w112:u32)
    n79 = feedback #1(u32 0 ("millisecond timer value")) -> (w113:u32)
    n80 = feedback-in #1(w112) -> ()
    n81 = Subtract(x=w112, y=w113) -> (x-y=→"HENES Loop Time":u32)
    n82 = local read "Stop"() -> (w110:bool)
  }
  n83 = while {
    shift-right: [w264] -> _
    shift-left: 0 ("Index(near vehicle)") -> [w263]
    stop <- w262 stop-if-true
    # "RPM을 100%로 환산(0~230PRM)"
    # "KHP→RPM"
    # "GPS Steer"
    n84 = case shown="\"Stanley Method\"" "Steer Selector" {
      tunnel: [w310 w343] -> w258
      tunnel: [w288 w311] -> w264
      tunnel: w263 -> [w293 w311]
      tunnel: [w291 w316] -> w260
      tunnel: [w292 w315] -> w259
      frame "Pure Pursuit", Default {
        # "가장 가까운 점 계산"
        # "Pure Pursuit"
        n85 = local read "True_Heading(deg)"() -> (w285:dbl)
        n86 = property on="Path_lat_arr" class="Arr (strict)"() -> ("Value"=w290:dbl[])  [unwired: 2 in, 2 out]
        n87 = property on="Path_long_arr" class="Arr (strict)"() -> ("Value"=w289:dbl[])  [unwired: 2 in, 2 out]
        n88 = local read "Path_Vel_arr"() -> (w294:dbl[])
        n89 = Index Array(array=w294, index=w293) -> (element=→"RDDF_Velocity":dbl)
        n90 = Index Array(array=w290, index=w293) -> (element=w292:dbl)
        n91 = Index Array(array=w289, index=w293) -> (element=w291:dbl)
        n92 = local read "UTM Y(N) INS"() -> (w287:dbl)
        n93 = local read "UTM X(E) INS"() -> (w286:dbl)
        n94 = Array Size(array=w289) -> (size(s)=w303:i32)
        n95 = To Long Integer(number=w303) -> (32bit integer=w302:i32)
        n96 = Subtract(x=w292, y=w287) -> (x-y=w309:dbl)
        n97 = Subtract(x=w291, y=w286) -> (x-y=w308:dbl)
        n98 = Square(x=w309) -> (x^2=w307:dbl)
        n99 = Square(x=w308) -> (x^2=w306:dbl)
        n100 = call "Pure Pursuit_New (Sub VI).vi"("x_lat_path"=w289, "L"=0.85, "y_long_path"=w290, "X_Current"=w287, "Y_Current"=w286, "Heading_Current"=w285, "#pnt"=w302, "WP no_pre"=0, "LAD"="Ld(m)") -> ("Steer_CMD(Deg)"=w298:dbl, "Index(near vehicle)"=w288:i32)  [unwired: 3 in, 2 out]
        n101 = Add(x=w307, y=w306) -> (x+y=w305:dbl)
        n102 = Square Root(x=w305) -> (sqrt(x)=→"Tracking_Err(m)":dbl)
        n103 = call "MultiNPointAverager.vi"("N point average"=3 ("WP no_pre"), "Data_input"=w298) -> ("숫자형"=w310:dbl)  [unwired: 9 in]
        n104 = Wait Until Next ms Multiple(millisecond multiple=u32 100 ("ms 배수")) -> ()  [unwired: 1 out]
      }
      frame "Stanley Method" {
        # "Stanley Method를 이용해 계산한 최적의 조향값 계산"
        # "차량 진행 방향"
        # "Stanley Method를 사용하기 위한 Heading Error 계산"
        # "라디안을 -pi~pi 사이로 정규화"
        # "라디안을 -pi~pi 사이로 정규화"
        # "경로상 가장 가까운 점과의 거리 계산\n경로상 왼쪽에 있으면 양수, 오른쪽에 있으면 음수"
        # "Heading Error 계산을 위해\n경로 상 가장  가까운 점의 방향을 계산"
        # "가장 가까운 점 계산"
        # "Stanley Method"
        n105 = local read "Path_long_arr"() -> (w341:dbl[])
        n106 = local read "Path_lat_arr"() -> (w340:dbl[])
        n107 = local read "UTM X(E) INS"() -> (w338:dbl)
        n108 = local read "UTM Y(N) INS"() -> (w339:dbl)
        n109 = for {
          tunnel: w338 -> [w356]
          tunnel: w339 -> [w355]
          tunnel: w340 -> [w347] mode=indexing
          tunnel: w341 -> [w348] mode=indexing
          tunnel: [w349] -> w342 mode=indexing
          # "Distance Calcualtor"
          n110 = Subtract(x=w356, y=w347) -> (x-y=w354:dbl)
          n111 = Subtract(x=w355, y=w348) -> (x-y=w353:dbl)
          n112 = Square(x=w354) -> (x^2=w352:dbl)
          n113 = Square(x=w353) -> (x^2=w351:dbl)
          n114 = Add(x=w352, y=w351) -> (x+y=w350:dbl)
          n115 = Square Root(x=w350) -> (sqrt(x)=w349:dbl)
        }
        n116 = Array Max & Min(array=w342) -> (min index (indices)=w313:i32)  [unwired: 3 out]
        n117 = local read "Path_long_arr"() -> (w332:dbl[])
        n118 = local read "Path_lat_arr"() -> (w333:dbl[])
        n119 = local read "UTM Y(N) INS"() -> (w336:dbl)
        n120 = local read "UTM X(E) INS"() -> (w337:dbl)
        n121 = Add(x=w313, y=2) -> (x+y=w312:i32)
        n122 = Add(x=w312, y=1) -> (x+y=w335:i32)
        n123 = Index Array(array=w333, index=w312) -> (element=w315:dbl)
        n124 = Index Array(array=w332, index=w312) -> (element=w316:dbl)
        n125 = Index Array(array=w333, index=w335) -> (element=w331:dbl)
        n126 = Index Array(array=w332, index=w335) -> (element=w330:dbl)
        n127 = call "CTECalculator.vi"("yp"=w336, "xi"=w315, "xp"=w337, "yi1"=w330, "xi1"=w331, "yi"=w316) -> ("CTE"=→"CTE":dbl)
        n128 = call "PathHeadingCalculator.vi"("yi1"=w330, "xi1"=w331, "yi"=w316, "xi"=w315) -> ("PathHeading"=w345:dbl)
        n129 = local read "True_Heading(deg)"() -> (w325:dbl)
        n130 = expression code="(x/180.0)*pi" ("degrees to radians")(w325) -> (w327:dbl)
        n131 = formula code="b = atan2(sin(a), cos(a));"("a"=w327) -> ("b"=w326:dbl)
        n132 = Subtract(x=w345, y=w326) -> (x-y=w328:dbl)
        n133 = formula code="b = atan2(sin(a), cos(a));"("a"=w328) -> ("b"=w344:dbl)
        n134 = local read "GPS_Speed(kph)"() -> (w324:dbl)
        n135 = local read "CTE"() -> (w320:dbl)
        n136 = Divide(x=w324, y=3.6) -> (x/y=w323:dbl)
        n137 = In Range and Coerce(upper limit=2.0, x=w323, lower limit=1.0) -> (coerced(x)=w322:dbl)  [unwired: 1 out]
        n138 = call "StanleyMethod.vi"("v(Velocity)m/s"=w322, "e(Cross-Track Err)m/s"=w320, "k(Gain)"="k(Gain)", "ψ(Heading Err)radian"=w344) -> ("δ(OutputSteer)degrees"=w343:dbl)  [unwired: 1 out]
        n139 = Wait Until Next ms Multiple(millisecond multiple=u32 100) -> ()  [unwired: 1 out]
      }
    }
    "xi" <- w259
    "yi" <- w260
    n140 = expression code="x/(0.00001*27*pi*60)"("Input_Spd(kph)") -> (w283:dbl)
    n141 = expression code="x*4.35*1.8"(w283) -> (→"Output_Spd_CMD(%)":dbl)
    n142 = local read "Y_long_path_Full"() -> (w280:dbl[])
    n143 = local read "X_lat_path_Full"() -> (w281:dbl[])
    n144 = local read "UTM Y(N) INS"() -> (w278:dbl)
    n145 = local read "Path_long_arr"() -> (w274:dbl[])
    n146 = local read "UTM X(E) INS"() -> (w279:dbl)
    n147 = local read "Path_lat_arr"() -> (w275:dbl[])
    n148 = In Range and Coerce(upper limit=20.0, x=w258, lower limit=-20.0) -> (coerced(x)=→"GPS_Steer_CMD(Deg)":dbl)  [unwired: 1 out]
    n149 = local read "xi"() -> (w273:dbl)
    n150 = local read "yi"() -> (w272:dbl)
    n151 = Build Array(w279) -> (w277:dbl[])
    n152 = Build Array(w278) -> (w276:dbl[])
    n153 = Build Array(w273) -> (w271:dbl[])
    n154 = Build Array(w272) -> (w270:dbl[])
    n155 = Bundle(w277, w276) -> (w269:cluster{dbl[], dbl[]})  [unwired: 1 in]
    n156 = Bundle(w271, w270) -> (w268:cluster{dbl[], dbl[]})  [unwired: 1 in]
    n157 = Bundle("X_lat_path_Full"=w281, "Y_long_path_Full"=w280) -> (w267:T7)  [unwired: 1 in]
    n158 = Bundle("Path_lat_arr"=w275, "Path_long_arr"=w274) -> (w266:T8)  [unwired: 1 in]
    n159 = Build Array(w269, w268, w267, w266) -> (→"GPS":T9)
    n160 = local read "Stop"() -> (w262:bool)
  }
  n161 = while {
    shift-right: [w365] -> _
    shift-left: _ -> [w366]
    tunnel: w42 -> [w363]
    tunnel: w38 -> [w358]
    tunnel: w40 -> [w360]
    tunnel: w41 -> [w359]
    tunnel: w39 -> [w357]
    stop <- w362 stop-if-true
    # "Near Point Finder"
    n162 = Wait Until Next ms Multiple(millisecond multiple=u32 50) -> ()  [unwired: 1 out]
    n163 = flat-sequence {
      tunnel: [w378] -> w364
      tunnel: w366 -> [w379]
      tunnel: w363 -> [w374]
      tunnel: w358 -> [w373]
      tunnel: w360 -> [w372]
      tunnel: w359 -> [w371]
      tunnel: w357 -> [w370]
      tunnel: [w404] -> w365
      tunnel: w364 -> [w404]
      frame #0 {
        n164 = local read "True_Heading(deg)"() -> (w367:dbl)
        n165 = local read "UTM Y(N) INS"() -> (w368:dbl)
        n166 = local read "UTM X(E) INS"() -> (w369:dbl)
        n167 = First Call?() -> (First Call?: T/F=w376:bool)
        n168 = Or(x=w376, y="Map Refresh") -> (x .or. y?=w377:bool)
        n169 = case shown="False" w377 {
          tunnel: w371 -> [w391 w402]
          tunnel: w372 -> [w392 w401]
          tunnel: w379 -> [w390 _]
          tunnel: w373 -> [w393 _]
          tunnel: w374 -> [w394 _]
          tunnel: [w395 w399] -> w378
          tunnel: w370 -> [w389 _]
          tunnel: w369 -> [w388 w398]
          tunnel: w368 -> [w387 w397]
          tunnel: w367 -> [_ w396]
          frame False {
            n170 = call "Local_Path_New_Stop(SubVI).vi"("x_lat_arr"=w391, "WP no_pre"=w390, "y_long_arr"=w392, "vel_arr"=w393, "x_lat_c"=w388, "y_long_c"=w387, "evt_arr"=w389, "# of pnt"=15) -> ("INDEX(Near Point)"=w386:i32, "Evt(Local)"=w383:dbl[], "Lat(Local)"=→"Path_lat_arr":dbl[], "Long(Local)"=→"Path_long_arr":dbl[], "Vel(Local)"=→"Path_Vel_arr":dbl[])  [unwired: 3 in]
            "WP_no." <- w386
            "Path_Evt_arr" <- w383
            n171 = Index Array(array=w383, index=w386) -> (element=→"Evt":dbl)
            n172 = Quotient & Remainder(x=w386, y=w394) -> (x-y*floor(x/y)=w395:i32)  [unwired: 1 out]
          }
          frame True {
            n173 = call "Local_Path_Second (SubVI).vi"("heading_deg"=w396, "heading_limit"=179.0, "y_long"=w397, "x_lat"=w398, "Y_long_path"=w401, "X_lat_path"=w402) -> ("Index(near vehicle)"=w399:i32)  [unwired: 1 out]
          }
        }
      }
      frame #1 {
        n174 = local write "Map Refresh"(FALSE ("Refresh")) -> ()
      }
    }
    n175 = local read "Stop"() -> (w362:bool)
    "X_lat_path_Full" <- w359
    "vel. path" <- w358
    "Y_long_path_Full" <- w360
    "Evt.Arr" <- w357
  }
  n176 = VISA Close(VISA resource name=w1, error in (no error)=w3) -> (error out=w2:errorcluster)
  n177 = property on="Stop" class="Bool (strict)"("Value"=w9) -> ()  [unwired: 2 in, 2 out]
  n178 = call <vilib>:"Clear Errors.vi"("error in (no error)"=w2) -> ()  [unwired: 5 in, 2 out]
  n179 = VISA Flush I/O Buffer(VISA resource name=w32, error in (no error)=w31) -> (VISA resource name out=w35:refnum<visa-resource-name>, error out=w36:errorcluster)  [unwired: 1 in]
  n180 = VISA Close(VISA resource name=w35, error in (no error)=w36) -> (error out=w30:errorcluster)
  n181 = call <vilib>:"Simple Error Handler.vi"("error in (no error)"=w30) -> ()  [unwired: 4 in, 5 out]
